vi "Safety_Check.vi"(1 "Adam Loop Count":i32, 2 "Ch Names":string[](array[string]), 3 "Values":dbl[](array[numeric]) format="%.2f") -> (0 "Scan comment":string)   [LabVIEW 2015]
uses:
  ADAM Client/Sub VIs/ADAM Controls/Update_scan_value.ctl
  Anemometry/Anemometry Sub Vis/Globals/Gas_management_global.vi
  ADAM_Global.vi
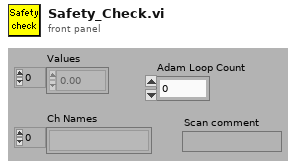
[diagram p1: front panel]
types:
  T1 = cluster{"Channel name":string, "Set value of A to":dbl, "Set value of B to":dbl, "Set value of C to":dbl, "Set value of D to":dbl}
  T2 = typedef "Update_scan_value.ctl" = cluster{"Channel Name":string, "New Value":dbl}
  T3 = enum16{"Append to Global", "Read Global then Clear"}
  T4 = enum16{"On", "Off", "Always On", "Always Off", "Delete"}
  T5 = typedef "LVDateTimeRec.ctl" = cluster{"fractional second":dbl, "second":i32, "minute":i32, "hour":i32, "day of month":i32, "month":i32, "year":i32, "day of week":i32, "day of year":i32, "DST":i32}
  T6 = cluster{"Channel name":string, "Set value of A to":dbl, "Set value of B to":dbl, "Set value of C to":dbl, "Set value of D to":dbl}[]
  T7 = typedef "Ch_description_ADAM.ctl" = cluster{"Ch Name":string, "Type":T8, "Function":T9, "Ch State":T10, "Calibration type":T11, "A":dbl, "B":dbl, "C":dbl, "D":dbl, "Comments":string, "Address":T12, "String":string, "Duty":u16}
  T8 = typedef "Module_type_ADAM.ctl" = string
  T9 = typedef "Function_ADAM.ctl" = enum16{"Analogue Input", "Digital Input", "Event counter", "Event rate", "Analogue Output", "Digital Output", "Relay Output"}
  T10 = typedef "Channel_State.ctl" = enum16{"On", "Off", "Always On", "Always Off"}
  T11 = typedef "Calib_type_ADAM.ctl" = enum16{"Raw", "Bx + A", "Cx^2 + Bx + A", "Dx^3 + Cx^2 + Bx + A", "In Band", "Hi-Tec Q", "Hi-Tec M_dot", "Text"}
  T12 = typedef "Address.ctl" = cluster{"Main":i32, "Ch.":i32, "Sub":i32, "Port Name":string}
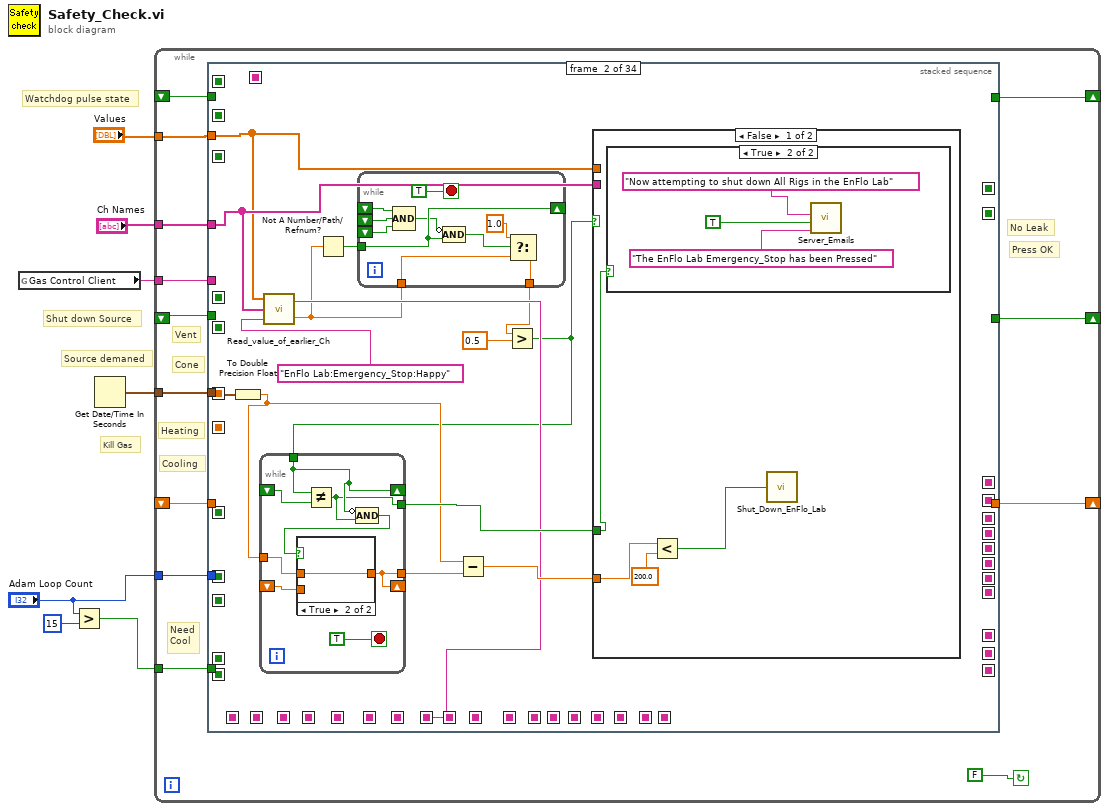
[diagram p0: block diagram]
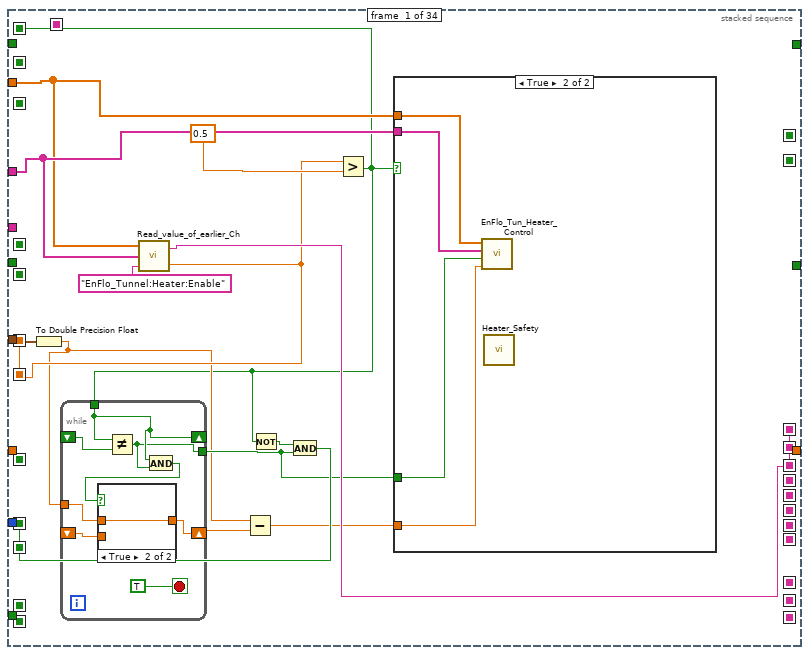
[diagram p2: hidden frame]
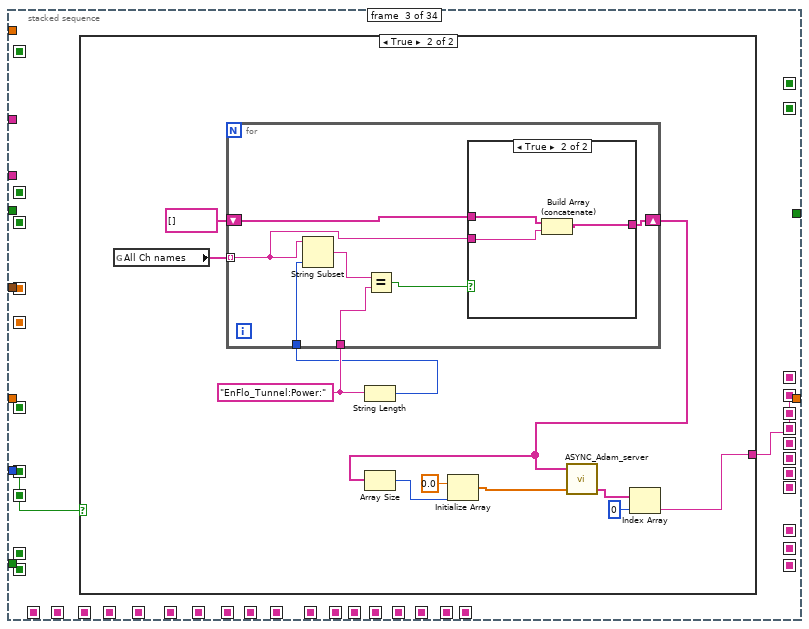
[diagram p8: hidden frame]
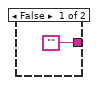
[diagram p9: hidden frame]
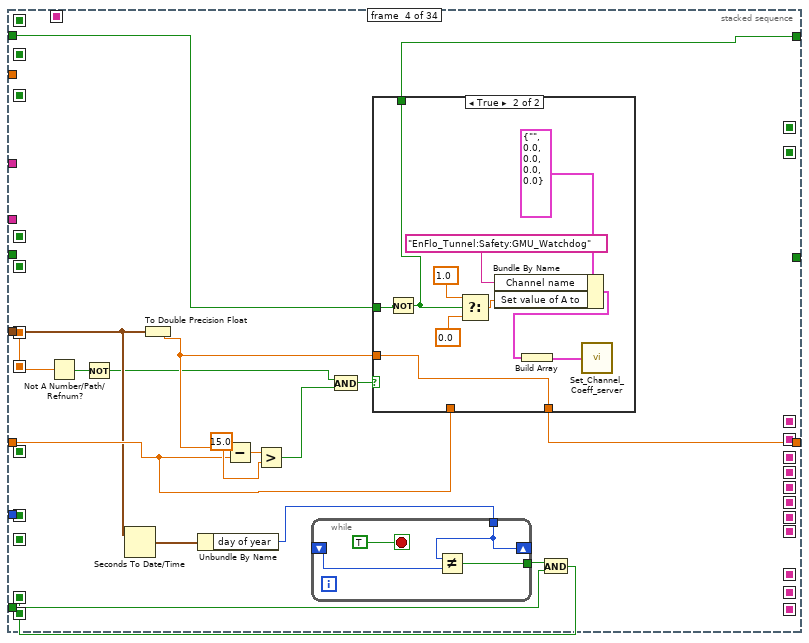
[diagram p11: hidden frame]
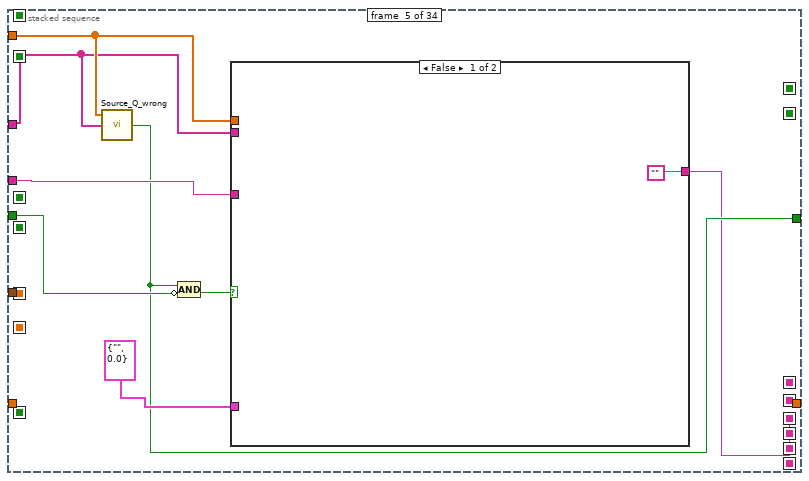
[diagram p13: hidden frame]
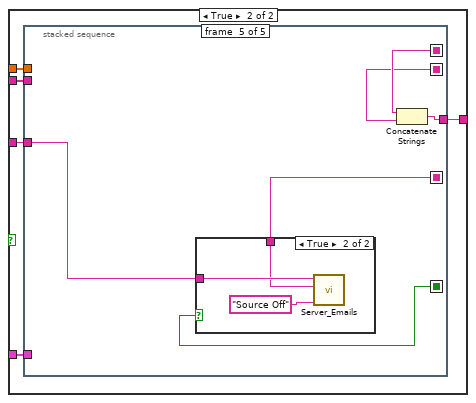
[diagram p14: hidden frame]
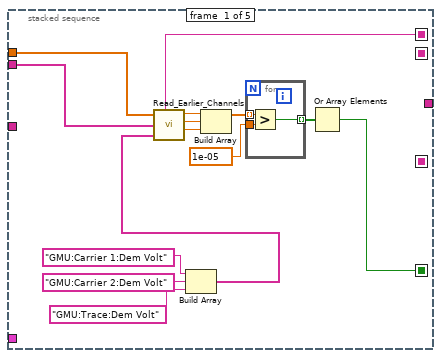
[diagram p15: hidden frame]
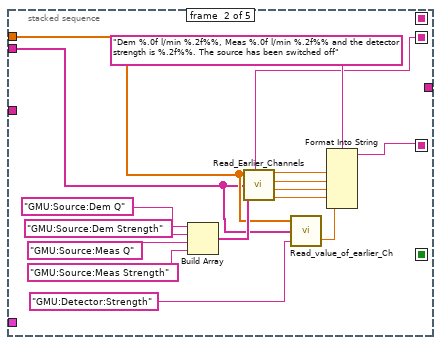
[diagram p16: hidden frame]
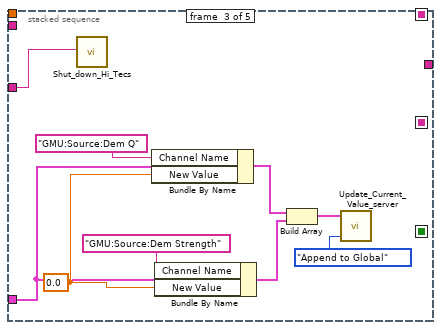
[diagram p17: hidden frame]
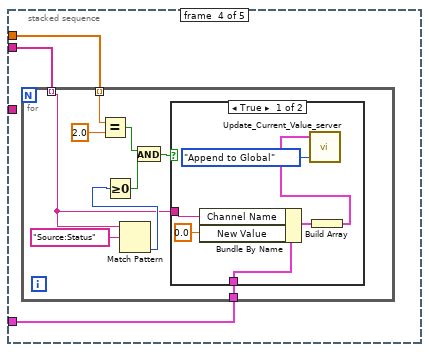
[diagram p18: hidden frame]
diagram:
  # "Shut down Source"
  # "Source demaned"
  # "Watchdog pulse state"
  # "Kill Gas"
  n1 = global read "Gas_management_global.vi" "Gas Control Client"() -> (w5:string)
  n2 = Greater?(x="Adam Loop Count", y=15) -> (0:w3:bool)
  n3 = Get Date/Time In Seconds() -> (seconds since 1Jan1904=w2:timestamp)
  n4 = while {
    shift-left: _ -> [w15]
    shift-right: [w14] -> _
    shift-left: _ -> [w17]
    shift-right: [w16] -> _
    tunnel: w5 -> [w19]
    tunnel: "Ch Names" -> [w20]
    tunnel: "Values" -> [w18]
    shift-right: [w12] -> _
    shift-left: _ -> [w11]
    tunnel: w3 -> [w10]
    tunnel: w2 -> [w9]
    tunnel: "Adam Loop Count" -> [w8]
    stop <- FALSE continue-if-true
    # "Need\nCool"
    # "Cooling"
    # "Heating"
    # "Cone"
    # "Vent"
    # "Press OK"
    # "No Leak"
    n5 = stacked-sequence {
      seq-local: [_ _ _ _ _ _ _ w272 _ _ _ _ _ _ _ _ _ _ _ _ _ _ _ _ _ _ _ _ _ _ _ _ _ _] -> [_ _ _ _ _ _ _ _ _ _ _ _ _ _ _ _ _ _ _ _ _ w692 _ _ _ _ _ _ _ _ _ _ _ _]
      seq-local: [w28 _ _ _ _ _ _ _ _ _ _ _ _ _ _ _ _ _ _ _ _ _ _ _ _ _ _ _ _ _ _ _ _ _] -> [_ _ w91 _ _ _ _ _ _ _ _ _ _ _ _ _ _ _ _ _ _ _ _ _ _ _ _ _ _ _ _ _ _ _]
      seq-local: [_ _ _ w121 _ _ _ _ _ _ _ _ _ _ _ _ _ _ _ _ _ _ _ _ _ _ _ _ _ _ _ _ _ _] -> [_ _ _ _ _ _ _ _ _ _ _ _ _ _ _ _ _ _ _ _ _ _ _ _ _ _ _ _ _ _ _ _ _ _]
      seq-local: [_ _ _ _ _ _ _ _ _ _ _ _ _ _ _ _ _ _ _ _ _ _ _ _ _ w822 _ _ _ _ _ _ _ _] -> [_ _ _ _ _ _ _ _ _ _ _ _ _ _ _ _ _ _ _ _ _ _ _ _ _ _ w834 _ _ _ _ _ _ _]
      seq-local: [_ _ _ _ _ _ _ _ _ _ _ _ _ _ _ _ _ _ _ _ _ _ _ _ _ _ w830 _ _ _ _ _ _ _] -> [_ _ _ _ _ _ _ _ _ _ _ _ _ _ _ _ _ _ _ _ _ _ _ _ _ _ _ _ _ _ _ w1016 _ _]
      seq-local: [w30 _ _ _ _ _ _ _ _ _ _ _ _ _ _ _ _ _ _ _ _ _ _ _ _ _ _ _ _ _ _ _ _ _] -> [_ _ _ _ _ _ _ _ _ _ _ _ _ _ _ _ _ _ _ _ _ _ _ _ _ _ _ _ _ _ _ _ _ w1096]
      seq-local: [_ _ w90 _ _ _ _ _ _ _ _ _ _ _ _ _ _ _ _ _ _ _ _ _ _ _ _ _ _ _ _ _ _ _] -> [_ _ _ _ _ _ _ _ _ _ _ _ _ _ _ _ _ _ _ _ _ _ _ _ _ _ _ _ _ _ _ _ _ w1095]
      seq-local: [_ _ _ _ w149 _ _ _ _ _ _ _ _ _ _ _ _ _ _ _ _ _ _ _ _ _ _ _ _ _ _ _ _ _] -> [_ _ _ _ _ _ _ _ _ _ _ _ _ _ _ _ _ _ _ _ _ _ _ _ _ _ _ _ _ _ _ _ _ w1094]
      seq-local: [_ _ _ _ _ w232 _ _ _ _ _ _ _ _ _ _ _ _ _ _ _ _ _ _ _ _ _ _ _ _ _ _ _ _] -> [_ _ _ _ _ _ _ _ _ _ _ _ _ _ _ _ _ _ _ _ _ _ _ _ _ _ _ _ _ _ _ _ _ w1093]
      seq-local: [_ _ _ _ _ _ w252 _ _ _ _ _ _ _ _ _ _ _ _ _ _ _ _ _ _ _ _ _ _ _ _ _ _ _] -> [_ _ _ _ _ _ _ _ _ _ _ _ _ _ _ _ _ _ _ _ _ _ _ _ _ _ _ _ _ _ _ _ _ w1092]
      seq-local: [_ _ _ _ _ _ _ w271 _ _ _ _ _ _ _ _ _ _ _ _ _ _ _ _ _ _ _ _ _ _ _ _ _ _] -> [_ _ _ _ _ _ _ _ _ _ _ _ _ _ _ _ _ _ _ _ _ _ _ _ _ _ _ _ _ _ _ _ _ w1091]
      seq-local: [_ _ _ _ _ _ _ _ _ _ _ w403 _ _ _ _ _ _ _ _ _ _ _ _ _ _ _ _ _ _ _ _ _ _] -> [_ _ _ _ _ _ _ _ _ _ _ _ _ _ _ _ _ _ _ _ _ _ _ _ _ _ _ _ _ _ _ _ _ w1090]
      seq-local: [_ _ _ _ _ _ _ _ _ _ _ _ w435 _ _ _ _ _ _ _ _ _ _ _ _ _ _ _ _ _ _ _ _ _] -> [_ _ _ _ _ _ _ _ _ _ _ _ _ _ _ _ _ _ _ _ _ _ _ _ _ _ _ _ _ _ _ _ _ w1081]
      seq-local: [_ _ _ _ _ _ _ _ _ _ _ _ _ _ _ _ _ w581 _ _ _ _ _ _ _ _ _ _ _ _ _ _ _ _] -> [_ _ _ _ _ _ _ _ _ _ _ _ _ _ _ _ _ _ _ _ _ _ _ _ _ _ _ _ _ _ _ _ _ w1080]
      seq-local: [_ _ _ _ _ _ _ _ _ _ _ _ _ _ _ _ _ _ _ _ _ w693 _ _ _ _ _ _ _ _ _ _ _ _] -> [_ _ _ _ _ _ _ _ _ _ _ _ _ _ _ _ _ _ _ _ _ _ _ _ _ _ _ _ _ _ _ _ _ w1083]
      seq-local: [_ _ _ _ _ _ _ _ _ _ _ _ _ _ _ _ _ _ _ _ _ _ w721 _ _ _ _ _ _ _ _ _ _ _] -> [_ _ _ _ _ _ _ _ _ _ _ _ _ _ _ _ _ _ _ _ _ _ _ _ _ _ _ _ _ _ _ _ _ w1084]
      seq-local: [_ _ _ _ _ _ _ _ _ _ _ _ _ _ _ _ _ _ _ _ _ _ _ _ _ w816 _ _ _ _ _ _ _ _] -> [_ _ _ _ _ _ _ _ _ _ _ _ _ _ _ _ _ _ _ _ _ _ _ _ _ _ _ _ _ _ _ _ _ w1085]
      seq-local: [_ _ _ _ _ _ _ _ _ _ _ _ _ _ _ _ _ _ _ _ _ _ _ _ _ _ w827 _ _ _ _ _ _ _] -> [_ _ _ _ _ _ _ _ _ _ _ _ _ _ _ _ _ _ _ _ _ _ _ _ _ _ _ _ _ _ _ _ _ w1086]
      seq-local: [_ _ _ _ _ _ _ _ _ _ _ _ _ w466 _ _ _ _ _ _ _ _ _ _ _ _ _ _ _ _ _ _ _ _] -> [_ _ _ _ _ _ _ _ _ _ _ _ _ _ _ _ _ _ _ _ _ _ _ _ _ _ _ _ _ _ _ _ _ w1087]
      seq-local: [_ _ _ _ _ _ _ _ _ _ _ _ _ _ _ _ _ _ _ _ _ _ _ _ _ _ _ _ _ _ w972 _ _ _] -> [_ _ _ _ _ _ _ _ _ _ _ _ _ _ _ _ _ _ _ _ _ _ _ _ _ _ _ _ _ _ _ _ _ w1088]
      seq-local: [_ _ _ _ _ _ _ _ _ _ _ _ _ _ _ _ _ _ _ _ _ _ _ _ _ _ _ _ _ _ _ w1014 _ _] -> [_ _ _ _ _ _ _ _ _ _ _ _ _ _ _ _ _ _ _ _ _ _ _ _ _ _ _ _ _ _ _ _ _ w1089]
      seq-local: [w29 _ _ _ _ _ _ _ _ _ _ _ _ _ _ _ _ _ _ _ _ _ _ _ _ _ _ _ _ _ _ _ _ _] -> [_ _ _ w119 _ _ _ _ _ _ _ _ _ _ _ _ _ _ _ _ _ _ _ _ _ _ _ w904 w931 _ _ _ _ _]
      seq-local: [_ _ _ _ _ _ _ _ w290 _ _ _ _ _ _ _ _ _ _ _ _ _ _ _ _ _ _ _ _ _ _ _ _ _] -> [_ _ _ _ _ _ _ _ _ _ _ _ _ _ _ _ _ _ _ _ _ w691 _ _ _ _ _ _ _ _ _ _ _ _]
      seq-local: [_ _ _ _ _ _ _ _ w289 _ _ _ _ _ _ _ _ _ _ _ _ _ _ _ _ _ _ _ _ _ _ _ _ _] -> [_ _ _ _ _ _ _ _ _ _ _ _ _ _ _ _ _ _ _ _ _ _ _ _ _ _ _ _ _ _ _ _ _ w1079]
      seq-local: [_ _ _ _ _ _ _ _ w288 _ _ _ _ _ _ _ _ _ _ _ _ _ _ _ _ _ _ _ _ _ _ _ _ _] -> [_ _ _ _ _ _ _ _ _ w317 w336 _ _ _ _ _ _ _ _ _ _ _ _ _ _ w817 w826 _ _ w957 _ _ _ _]
      seq-local: [_ _ _ _ _ _ _ _ _ _ w333 _ _ _ _ _ _ _ _ _ _ _ _ _ _ _ _ _ _ _ _ _ _ _] -> [_ _ _ _ _ _ _ _ _ _ _ _ _ _ _ _ _ _ _ _ _ _ _ _ _ _ _ _ _ _ _ _ _ w1077]
      seq-local: [_ _ _ _ _ _ _ _ _ _ _ _ _ _ _ _ w535 _ _ _ _ _ _ _ _ _ _ _ _ _ _ _ _ _] -> [_ _ _ _ _ _ _ _ _ _ _ _ _ _ _ _ _ _ _ _ _ _ _ _ _ _ _ _ _ _ _ _ _ w1078]
      seq-local: [_ _ _ _ _ _ _ _ _ _ _ _ _ _ _ _ _ _ _ _ _ _ _ _ w784 _ _ _ _ _ _ _ _ _] -> [_ _ _ _ _ _ _ _ _ _ _ _ _ _ _ _ _ _ _ _ _ _ _ _ _ _ _ _ _ _ _ _ _ w1076]
      seq-local: [_ _ _ _ _ _ _ _ _ _ _ _ _ _ w494 _ _ _ _ _ _ _ _ _ _ _ _ _ _ _ _ _ _ _] -> [_ _ _ _ _ _ _ _ _ _ _ _ _ _ _ _ _ _ _ _ _ _ _ _ _ _ _ _ _ _ _ _ _ w1075]
      seq-local: [_ w55 _ _ _ _ _ _ _ _ _ _ _ _ _ _ _ _ _ _ _ _ _ _ _ _ _ _ _ _ _ _ _ _] -> [_ _ _ _ _ _ _ _ _ _ _ _ _ _ _ _ _ _ _ _ _ _ _ _ _ _ _ _ _ _ _ _ _ w1074]
      seq-local: [_ _ _ _ _ _ _ _ _ _ _ _ _ _ _ _ _ _ _ _ _ _ _ _ _ _ _ _ _ _ _ _ w1040 _] -> [_ _ _ _ _ _ _ _ _ _ _ _ _ _ _ _ _ _ _ _ _ _ _ _ _ _ _ _ _ _ _ _ _ w1073]
      seq-local: [_ _ _ _ _ _ _ _ _ _ _ _ _ _ _ _ _ _ w603 _ _ _ _ _ _ _ _ _ _ _ _ _ _ _] -> [_ _ _ _ _ _ _ _ _ _ _ _ _ _ _ _ _ _ _ _ _ _ _ _ _ _ _ _ _ _ _ _ _ w1071]
      seq-local: [_ _ _ _ _ _ _ _ _ _ _ _ _ _ _ _ _ _ _ _ w671 _ _ _ _ _ _ _ _ _ _ _ _ _] -> [_ _ _ _ _ _ _ _ _ _ _ _ _ _ _ _ _ _ _ _ _ _ _ _ _ _ _ _ _ _ _ _ _ w1072]
      seq-local: [w21 _ _ _ _ _ _ _ _ _ _ _ _ _ _ _ _ _ _ _ _ _ _ _ _ _ _ _ _ _ _ _ _ _] -> [_ _ _ _ _ _ _ _ _ _ _ _ _ _ _ _ _ _ _ _ _ _ w720 w741 _ _ _ _ _ _ _ _ _ _]
      seq-local: [_ _ _ _ _ _ _ _ _ _ _ _ _ _ _ _ _ _ _ _ _ _ _ w739 _ _ _ _ _ _ _ _ _ _] -> [_ _ _ _ _ _ _ _ _ _ _ _ _ _ _ _ _ _ _ _ _ _ _ _ _ _ _ _ _ _ _ _ _ w1070]
      seq-local: [_ _ _ _ _ _ _ _ _ _ _ _ _ _ _ _ _ _ _ _ _ _ _ _ _ _ _ _ _ w956 _ _ _ _] -> [_ _ _ _ _ _ _ _ _ _ _ _ _ _ _ _ _ _ _ _ _ _ _ _ _ _ _ _ _ _ _ _ _ w1069]
      seq-local: [_ _ _ _ _ _ _ _ _ _ _ _ _ w455 _ _ _ _ _ _ _ _ _ _ _ _ _ _ _ _ _ _ _ _] -> [_ _ _ _ _ _ _ _ _ _ _ _ _ _ _ w515 _ _ _ _ _ _ _ _ _ _ _ _ _ _ _ _ _ _]
      seq-local: [_ _ _ _ _ _ _ _ _ _ _ _ _ _ w493 _ _ _ _ _ _ _ _ _ _ _ _ _ _ _ _ _ _ _] -> [_ _ _ _ _ _ _ _ _ _ _ _ _ _ _ w516 _ _ _ _ _ _ _ _ _ _ _ _ _ _ _ _ _ _]
      seq-local: [_ _ _ _ _ _ _ _ _ _ _ _ _ _ _ _ _ _ _ _ _ _ _ _ _ _ w825 _ _ _ _ _ _ _] -> [_ _ _ _ _ _ _ _ _ _ _ _ _ _ _ _ _ _ _ _ _ _ _ _ _ _ _ w902 w921 _ _ _ _ _]
      seq-local: [_ _ _ _ _ _ _ _ _ _ _ _ _ _ _ _ _ _ _ _ _ _ _ _ _ _ _ w896 _ _ _ _ _ _] -> [_ _ _ _ _ _ _ _ _ _ _ _ _ _ _ _ _ _ _ _ _ _ _ _ _ _ _ _ _ _ _ _ _ w1068]
      seq-local: [_ _ _ _ _ _ _ _ _ _ _ _ _ _ _ _ _ _ _ _ _ _ _ _ _ _ _ _ w922 _ _ _ _ _] -> [_ _ _ _ _ _ _ _ _ _ _ _ _ _ _ _ _ _ _ _ _ _ _ _ _ _ _ _ _ _ _ _ _ w1067]
      seq-local: [_ _ _ _ _ _ _ _ _ w318 _ _ _ _ _ _ _ _ _ _ _ _ _ _ _ _ _ _ _ _ _ _ _ _] -> [_ _ _ _ _ _ _ _ _ _ w332 _ _ _ _ _ _ _ _ _ _ _ _ _ _ _ _ _ _ _ _ _ _ _]
      seq-local: [_ _ _ _ _ _ _ _ _ _ _ _ _ _ _ _ _ _ w602 _ _ _ _ _ _ _ _ _ _ _ _ _ _ _] -> [_ _ _ _ _ _ _ _ _ _ _ _ _ _ _ _ _ _ _ w641 _ _ _ _ _ _ _ _ _ _ _ _ _ _]
      seq-local: [_ _ _ _ _ _ _ _ _ _ _ _ _ _ _ _ _ _ _ w635 _ _ _ _ _ _ _ _ _ _ _ _ _ _] -> [_ _ _ _ _ _ _ _ _ _ _ _ _ _ _ _ _ _ _ _ _ _ _ _ _ _ _ _ _ _ _ _ _ w1066]
      tunnel: w20 -> [w32 w61 _ _ w151 w239 w254 w273 w291 w319 w334 w404 w436 w465 w495 _ w536 w583 w605 w647 w673 w694 w725 w745 w778 w820 w835 w889 _ _ w975 _ _ _]
      tunnel: w19 -> [_ _ _ _ w156 _ w253 _ _ _ _ _ _ _ _ _ _ _ _ _ _ _ _ _ _ _ _ _ _ _ _ _ _ _]
      tunnel: w18 -> [w31 w60 _ _ w152 w235 w255 w274 w292 w320 w335 w405 w437 w463 w496 _ w537 w584 w606 w648 w674 w695 w726 w746 w777 w821 w836 w890 _ _ w976 _ _ _]
      tunnel: w17 -> [_ _ _ w132 _ _ _ _ _ _ _ _ _ _ _ _ _ _ _ _ _ _ _ _ _ _ _ _ _ _ _ _ _ _]
      tunnel: [_ _ _ w131 _ _ _ _ _ _ _ _ _ _ _ _ _ _ _ _ _ _ _ _ _ _ _ _ _ _ _ _ _ _] -> w16
      tunnel: w15 -> [_ _ _ _ w155 _ _ _ _ _ _ _ _ _ _ _ _ _ _ _ _ _ _ _ _ _ _ _ _ _ _ _ _ _]
      tunnel: [_ _ _ _ w150 _ _ _ _ _ _ _ _ _ _ _ _ _ _ _ _ _ _ _ _ _ _ _ _ _ _ _ _ _] -> w14
      tunnel: [_ _ _ w130 _ _ _ _ _ _ _ _ _ _ _ _ _ _ _ _ _ _ _ _ _ _ _ _ _ _ _ _ _ _] -> w12
      tunnel: w11 -> [_ _ _ w126 _ _ _ _ _ _ _ _ _ _ _ _ _ _ _ _ _ _ _ _ _ _ _ _ _ _ _ _ _ _]
      tunnel: w10 -> [_ _ _ w122 _ _ _ _ _ _ _ _ _ w467 _ _ w533 w582 w604 w645 w672 _ _ _ _ _ w831 w897 w927 w955 _ w1015 _ _]
      tunnel: w9 -> [w25 w58 _ w120 _ _ _ _ _ _ _ _ _ _ _ _ w534 _ _ _ _ _ _ _ _ _ _ _ _ _ _ _ _ _]
      tunnel: w8 -> [_ _ _ _ _ _ _ _ _ _ _ _ _ _ _ _ _ _ _ _ _ _ _ _ _ _ _ _ _ _ _ _ w1052 _]
      frame #0 {
        n6 = To Double Precision Float(number=w25) -> (double precision float=w24:dbl)
        n7 = call "Read_value_of_earlier_Ch.vi"("Desired Ch to Read"="EnFlo_Tunnel:Heater:Enable", "Ch names"=w32, "Present scan array"=w31) -> ("Value"=w29:dbl, "Scan comment"=w30:string)  [unwired: 1 in]
        n8 = Greater?(x=w29, y=0.5) -> (0:w21:bool)
        n9 = while {
          shift-right: [w40] -> _
          shift-left: _ -> [w42]
          tunnel: w21 -> [w40]
          tunnel: [w39] -> w26
          shift-right: [w37] -> w23
          shift-left: _ -> [w35]
          tunnel: w24 -> [w36]
          stop <- TRUE stop-if-true
          n10 = Not Equal?(x=w40, y=w42) -> (x != y?=w39:bool)
          n11 = And(x=w40, y=w39) -> (x .and. y?=w38:bool)
          n12 = case shown="True" w38 {
            tunnel: [w43 w44] -> w37
            tunnel: w36 -> [_ w44]
            tunnel: w35 -> [w43 _]
            frame False {
            }
            frame True {
            }
          }
        }
        n13 = Subtract(x=w24, y=w23) -> (x-y=w22:dbl)
        n14 = Not(x=w21) -> (.not. x?=w27:bool)
        n15 = And(x=w27, y=w26) -> (x .and. y?=w28:bool)
        n16 = case shown="True" w21 {
          tunnel: w31 -> [_ w48]
          tunnel: w32 -> [_ w47]
          tunnel: w26 -> [_ w46]
          tunnel: w22 -> [_ w45]
          frame False {
          }
          frame True {
            n17 = call "EnFlo_Tun_Heater_Control.vi"("Heaters Enabled time (s)"=w45, "Heaters Just Enabled"=w46, "Ch Names"=w47, "Values"=w48) -> ()  [unwired: 1 in]
            n18 = call "Heater_Safety.vi"() -> ()  [unwired: 3 in, 5 out]
          }
        }
      }
      frame #1 {
        n19 = To Double Precision Float(number=w58) -> (double precision float=w57:dbl)
        n20 = call "Read_value_of_earlier_Ch.vi"("Desired Ch to Read"="EnFlo Lab:Emergency_Stop:Happy", "Ch names"=w61, "Present scan array"=w60) -> ("Value"=w53:dbl, "Scan comment"=w55:string)  [unwired: 1 in]
        n21 = Not A Number/Path/Refnum?(number/path/refnum=w53) -> (NaN/Path/Refnum?=w52:bool)
        n22 = while {
          tunnel: w53 -> [w65]
          shift-right: [w69] -> _
          shift-left: _ -> [w72]
          tunnel: w52 -> [w69]
          shift-left: _ -> [w71]
          shift-left: _ -> [w70]
          tunnel: [w64] -> w49
          stop <- TRUE stop-if-true
          n23 = Compound Arithmetic op=AND(w72, w71, w70) -> (w68:bool)
          n24 = Compound Arithmetic op=AND(invert w68, w69) -> (w67:bool)
          n25 = Select(t=1.0, s=w67, f=w65) -> (s? t:f=w64:dbl)
        }
        n26 = Greater?(x=w49, y=0.5) -> (0:w50:bool)
        n27 = while {
          shift-right: [w78] -> _
          shift-left: _ -> [w80]
          tunnel: w50 -> [w78]
          tunnel: [w77] -> w59
          shift-right: [w73] -> _
          shift-left: _ -> [w74]
          tunnel: w57 -> [w75]
          tunnel: [w73] -> w54
          stop <- TRUE stop-if-true
          n28 = Not Equal?(x=w78, y=w80) -> (x != y?=w77:bool)
          n29 = Compound Arithmetic op=AND(invert w78, w77) -> (w76:bool)
          n30 = case shown="True" w76 {
            tunnel: [w81 w82] -> w73
            tunnel: w75 -> [_ w82]
            tunnel: w74 -> [w81 _]
            frame False {
            }
            frame True {
            }
          }
        }
        n31 = Subtract(x=w57, y=w54) -> (x-y=w56:dbl)
        n32 = case shown="False" w50 {
          tunnel: w60 -> [_ _]
          tunnel: w61 -> [_ _]
          tunnel: w59 -> [w84 _]
          tunnel: w56 -> [w86 _]
          frame False {
            n33 = case shown="True" w84 {
              frame False {
              }
              frame True {
                n34 = call "Server_Emails.vi"("Message"="Now attempting to shut down All Rigs in the EnFlo Lab", "Contact All clients?"=TRUE, "Subject"="The EnFlo Lab Emergency_Stop has been Pressed") -> ()  [unwired: 2 in, 3 out]
              }
            }
            n35 = Less?(x=w86, y=200.0) -> (x < y?=w83:bool)
            n36 = call "Shut_Down_EnFlo_Lab.vi"("Initial Shutdown"=w83) -> ()
          }
          frame True {
          }
        }
      }
      frame #2 {
        n37 = case shown="True" w91 {
          tunnel: ["" w94] -> w90
          frame False {
          }
          frame True {
            w103 = "EnFlo_Tunnel:Power:"
            n38 = global read "ADAM_Global.vi" "All Ch names"() -> (w93:string[])
            n39 = String Length(string=w103) -> (length=w102:i32)
            n40 = for {
              shift-right: [w105] -> w98
              shift-left: string[] [] -> [w106]
              tunnel: w93 -> [w109] mode=indexing
              tunnel: w102 -> [w110]
              tunnel: w103 -> [w107]
              n41 = String Subset(string=w109, length (rest)=w110) -> (substring=w108:string)  [unwired: 1 out]
              n42 = Equal?(x=w108, y=w107) -> (x = y?=w104:bool)
              n43 = case shown="True" w104 {
                tunnel: w109 -> [_ w114]
                tunnel: w106 -> [w111 w112]
                tunnel: [w111 w113] -> w105
                frame False {
                }
                frame True {
                  n44 = Build Array (concatenate)(w112, w114) -> (w113:string[])
                }
              }
            }
            n45 = Array Size(array=w98) -> (size(s)=w99:i32)
            n46 = Initialize Array(0.0 ("element"), w99) -> (w97:dbl[])
            n47 = call "ASYNC_Adam_server.vi"("Values"=w97, "Channel Names"=w98) -> ("Scan Comments"=w96:string[])  [unwired: 1 in, 2 out]
            n48 = Index Array(array=w96, index=0) -> (element=w94:string)
          }
        }
      }
      frame #3 {
        n49 = Not A Number/Path/Refnum?(number/path/refnum=w119) -> (NaN/Path/Refnum?=w118:bool)
        n50 = Not(x=w118) -> (.not. x?=w116:bool)
        n51 = Seconds To Date/Time(time stamp (now)=w120) -> (date time rec=w125:T5)  [unwired: 1 in]
        n52 = To Double Precision Float(number=w120) -> (double precision float=w129:dbl)
        n53 = Unbundle By Name(w125) -> ("day of year"=w124:i32)
        n54 = Subtract(x=w129, y=w126) -> (x-y=w128:dbl)
        n55 = Greater?(x=w128, y=15.0) -> (0:w117:bool)
        n56 = while {
          shift-right: [w136] -> _
          shift-left: _ -> [w135]
          tunnel: w124 -> [w136]
          tunnel: [w134] -> w123
          stop <- TRUE stop-if-true
          n57 = Not Equal?(x=w136, y=w135) -> (x != y?=w134:bool)
        }
        n58 = And(x=w116, y=w117) -> (x .and. y?=w115:bool)
        n59 = case shown="True" w115 {
          tunnel: w132 -> [w137 w141]
          tunnel: [w137 w140] -> w131
          tunnel: [w138 w139] -> w130
          tunnel: w129 -> [_ w139]
          tunnel: w126 -> [w138 _]
          frame False {
          }
          frame True {
            n60 = Not(x=w141) -> (.not. x?=w140:bool)
            n61 = Select(t=1.0 ("Suction"), s=w140, f=0.0 ("Suction")) -> (s? t:f=w144:dbl)
            n62 = Bundle By Name(cluster=T1 {"Channel name"="", "Set value of A to"=0.0, "Set value of B to"=0.0, "Set value of C to"=0.0, "Set value of D to"=0.0}, "Channel name"="EnFlo_Tunnel:Safety:GMU_Watchdog" ("Desired Ch to Read"), "Set value of A to"=w144) -> (w148:T1)
            n63 = Build Array(w148) -> (w143:T6)
            n64 = call "Set_Channel_Coeff_server.vi"("Set Array"=w143) -> ()
          }
        }
        n65 = And(x=w123, y=w122) -> (x .and. y?=w121:bool)
      }
      frame #4 {
        n66 = call "Source_Q_wrong.vi"("Ch Names"=w151, "Values"=w152) -> ("Gas Error?"=w150:bool)  [unwired: 1 out]
        n67 = Compound Arithmetic op=AND(w150, invert w155) -> (w154:bool)
        n68 = case shown="False" w154 {
          tunnel: w156 -> [_ w162]
          tunnel: w152 -> [_ w161]
          tunnel: w151 -> [_ w160]
          tunnel: T2 {"Channel Name"="", "New Value"=0.0} ("Update Scan Value Cluster") -> [_ w159]
          tunnel: ["" w158] -> w149
          frame False {
          }
          frame True {
            n69 = stacked-sequence {
              seq-local: [_ w194 _ _ _] -> [_ _ _ _ w227]
              seq-local: [w164 _ _ _ _] -> [_ _ _ _ w226]
              seq-local: [w163 _ _ _ _] -> [_ _ _ _ w225]
              seq-local: [_ w180 _ _ _] -> [_ _ _ _ w224]
              tunnel: w162 -> [_ _ w197 _ w228]
              tunnel: w161 -> [w174 w184 _ w206 _]
              tunnel: w160 -> [w175 w183 _ w207 _]
              tunnel: w159 -> [_ _ w196 w205 _]
              tunnel: [_ _ _ _ w223] -> w158
              frame #0 {
                n70 = Build Array("GMU:Carrier 1:Dem Volt", "GMU:Carrier 2:Dem Volt", "GMU:Trace:Dem Volt") -> (w176:string[])
                n71 = call "Read_Earlier_Channels.vi"("Present scan array"=w174, "Ch names"=w175, "Desired Channels"=w176) -> ("Scan comments"=w163:string, "Index 0"=w170:dbl, "Index 1"=w169:dbl, "Index 2"=w168:dbl)  [unwired: 2 out]
                n72 = Build Array(w170, w169, w168) -> (w167:dbl[])
                n73 = for {
                  tunnel: w167 -> [w179] mode=indexing
                  tunnel: 1e-05 -> [w178]
                  tunnel: [w177] -> w165 mode=indexing
                  n74 = Greater?(x=w179, y=w178) -> (0:w177:bool)
                }
                n75 = Or Array Elements(Boolean array=w165) -> (logical OR=w164:bool)
              }
              frame #1 {
                n76 = Build Array("GMU:Source:Dem Q", "GMU:Source:Dem Strength", "GMU:Source:Meas Q", "GMU:Source:Meas Strength") -> (w189:string[])
                n77 = call "Read_Earlier_Channels.vi"("Present scan array"=w184, "Ch names"=w183, "Desired Channels"=w189) -> ("Scan comments"=w180:string, "Index 0"=w188:dbl, "Index 1"=w187:dbl, "Index 2"=w186:dbl, "Index 3"=w185:dbl)  [unwired: 1 out]
                n78 = call "Read_value_of_earlier_Ch.vi"("Desired Ch to Read"="GMU:Detector:Strength", "Ch names"=w183, "Present scan array"=w184) -> ("Value"=w181:dbl)  [unwired: 1 in, 1 out]
                n79 = Format Into String(format string="Dem %.0f l/min %.2f%%, Meas %.0f l/min %.2f%% and the detector strength is %.2f%%. The source has been switched off" ("Format String"), w188, w187, w186, w185, w181) -> (resulting string=w194:string)  [unwired: 2 in, 1 out]
              }
              frame #2 {
                w198 = 0.0 ("Bundle Element")
                n80 = call "Shut_down_Hi_Tecs.vi"("Client Name"=w197) -> ()  [unwired: 6 out]
                n81 = Bundle By Name(cluster=w196, "Channel Name"="GMU:Source:Dem Q", "New Value"=w198) -> (w203:T2)
                n82 = Bundle By Name(cluster=w196, "Channel Name"="GMU:Source:Dem Strength", "New Value"=w198) -> (w204:T2)
                n83 = Build Array(w203, w204) -> (w200:T2[])
                n84 = call "Update_Current_Value_server.vi"("Mode"=T3."Append to Global", "Update array in"=w200) -> ()  [unwired: 1 in, 1 out]
              }
              frame #3 {
                n85 = for {
                  tunnel: w207 -> [w208] mode=indexing
                  tunnel: w206 -> [w214] mode=indexing
                  tunnel: w205 -> [w209]
                  n86 = Equal?(x=w214, y=2.0) -> (x = y?=w211:bool)
                  n87 = Match Pattern(string=w208, regular expression="Source:Status") -> (offset past match=w215:i32)  [unwired: 4 out]
                  n88 = Greater Or Equal To 0?(x=w215) -> (x >= 0?=w212:bool)
                  n89 = And(x=w211, y=w212) -> (x .and. y?=w210:bool)
                  n90 = case shown="True" w210 {
                    tunnel: w209 -> [w222 _]
                    tunnel: w208 -> [w221 _]
                    frame True {
                      n91 = Bundle By Name(cluster=w222, "Channel Name"=w221, "New Value"=0.0) -> (w219:T2)
                      n92 = Build Array(w219) -> (w218:T2[])
                      n93 = call "Update_Current_Value_server.vi"("Mode"=T3."Append to Global", "Update array in"=w218) -> ()  [unwired: 1 in, 1 out]
                    }
                    frame False {
                    }
                  }
                }
              }
              frame #4 {
                n94 = case shown="True" w226 {
                  tunnel: w228 -> [_ w231]
                  tunnel: w227 -> [_ w230]
                  frame False {
                  }
                  frame True {
                    n95 = call "Server_Emails.vi"("Client Name Contains"=w231, "Message"=w230, "Subject"="Source Off") -> ()  [unwired: 2 in, 3 out]
                  }
                }
                n96 = Concatenate Strings(w225, w224) -> (w223:string)
              }
            }
          }
        }
      }
      frame #5 {
        n97 = global read "ADAM_Global.vi" "Program Hung Clients"() -> (w240:string[])
        n98 = for {
          tunnel: w240 -> [w249] mode=indexing
          tunnel: w235 -> [w251]
          tunnel: w239 -> [w250]
          tunnel: [w247] -> w238 mode=indexing
          tunnel: [w244] -> w237 mode=indexing
          shift-right: [w242] -> w232
          shift-left: "" -> [w243]
          n99 = call "Split_Ch_name.vi"("Ch name"=w249) -> ("Low level"=w246:string)  [unwired: 2 out]
          n100 = call "Shut_Down_Client_Demands.vi"("Ch Names"=w250, "Values"=w251, "Client Name"=w249) -> ("Comments"=w241:string)
          n101 = Concatenate Strings(w243, w241) -> (w242:string)
          n102 = Concatenate Strings(w246, ":Source:Status") -> (w247:string)
          n103 = Concatenate Strings(w246, ":Program:Sync") -> (w244:string)
        }
        n104 = Build Array (concatenate)(w238, w237) -> (w236:string[])
        n105 = call "Cntrl_Ch_Status_low.vi"("Mode"=T4."Delete", "Channel names"=w236) -> ()  [unwired: 1 out]
      }
      frame #6 {
        n106 = while {
          tunnel: w255 -> [w267]
          tunnel: w254 -> [w266]
          shift-right: [w261] -> _
          shift-left: _ -> [w262]
          tunnel: w253 -> [w259]
          tunnel: [w257] -> w252
          stop <- FALSE continue-if-true
          n107 = call "Read_value_of_earlier_Ch.vi"("Desired Ch to Read"="GMU:Detector:Happy", "Ch names"=w266, "Present scan array"=w267) -> ("Value"=w264:dbl, "Scan comment"=w257:string)  [unwired: 1 in]
          n108 = Greater?(x=w264, y=0.5) -> (0:w261:bool)
          n109 = Compound Arithmetic op=AND(invert w261, w262) -> (w260:bool)
          n110 = case shown="True" w260 {
            tunnel: w259 -> [_ w269]
            frame False {
            }
            frame True {
              n111 = call "Server_Emails.vi"("Client Name Contains"=w269, "Message"="The GMU Gas detector IR2100 is unhappy. Please check concentrations etc. This will have turned off the gases from the outside bottle store.  You will need to repress the blue gas button after clearing the fault by purging the source with carrier gas only.", "Subject"="GMU Gas Detector Unhappy") -> ()  [unwired: 2 in, 3 out]
            }
          }
        }
        n112 = global write "ADAM_Global.vi" "Program Hung Clients"(string[] [] ("Program Hung Clients")) -> ()
      }
      frame #7 {
        n113 = while {
          tunnel: w274 -> [w284]
          tunnel: w273 -> [w283]
          shift-right: [w278] -> w272
          shift-left: _ -> [w279]
          tunnel: [w275] -> w271
          stop <- FALSE continue-if-true
          n114 = call "Read_value_of_earlier_Ch.vi"("Desired Ch to Read"="EnFlo Lab:Leak_Detector:Happy", "Ch names"=w283, "Present scan array"=w284) -> ("Value"=w281:dbl, "Scan comment"=w275:string)  [unwired: 1 in]
          n115 = Greater?(x=w281, y=0.5) -> (0:w278:bool)
          n116 = Compound Arithmetic op=AND(invert w278, w279) -> (w277:bool)
          n117 = case shown="True" w277 {
            frame False {
            }
            frame True {
              n118 = call "Server_Emails.vi"("Client Name Contains"="EnFlo_Tunnel", "Message"="The leak detector is indicating a leak under the Enflo Tunnel. The chiller pumps should automaticaly be turned off and the cooling circuit isolated from the  University Chilled water system. The heaters should also have been disabled.", "Subject"="Leak Detected under EnFlo Tunnel") -> ()  [unwired: 2 in, 3 out]
            }
          }
        }
      }
      frame #8 {
        n119 = while {
          tunnel: w292 -> [w298]
          tunnel: w291 -> [w297]
          shift-right: [w309] -> w290
          shift-left: _ -> [w310]
          tunnel: [w301] -> w289
          tunnel: [w293] -> w288
          stop <- FALSE continue-if-true
          n120 = call "Read_value_of_earlier_Ch.vi"("Desired Ch to Read"="EnFlo_Tunnel:Chiller_Pump:Enable", "Ch names"=w297, "Present scan array"=w298) -> ("Value"=w304:dbl, "Scan comment"=w302:string)  [unwired: 1 in]
          n121 = call "Read_value_of_earlier_Ch.vi"("Desired Ch to Read"="EnFlo_Tunnel:Chilled Water:Pressure_OK", "Ch names"=w297, "Present scan array"=w298) -> ("Value"=w312:dbl, "Scan comment"=w303:string)  [unwired: 1 in]
          n122 = call "Read_value_of_earlier_Ch.vi"("Desired Ch to Read"="EnFlo_Tunnel:Chiller_Pump:Running", "Ch names"=w297, "Present scan array"=w298) -> ("Value"=w295:dbl, "Scan comment"=w294:string)  [unwired: 1 in]
          n123 = Greater?(x=w312, y=0.5) -> (0:w309:bool)
          n124 = Greater?(x=w304, y=0.5) -> (0:w300:bool)
          n125 = Compound Arithmetic op=AND(invert w309, w310, w300) -> (w308:bool)
          n126 = case shown="True" w308 {
            frame False {
            }
            frame True {
              n127 = call "Server_Emails.vi"("Client Name Contains"="EnFlo_Tunnel", "Message"="The pressure in the chilled water  for the Enflo Tunnel has tripped the system. The chiller pumps should automaticaly be turned off and the cooling circuit isolated from the  University Chilled water system. The heaters should also have been disabled.", "Subject"="EnFlo Chilled Water Overpressure Trip") -> ()  [unwired: 2 in, 3 out]
            }
          }
          n128 = Greater?(x=w295, y=0.5) -> (0:w293:bool)
          n129 = Concatenate Strings(w302, w303, w294) -> (w301:string)
        }
      }
      frame #9 {
        n130 = case shown="True" w317 {
          tunnel: w320 -> [_ w328]
          tunnel: w319 -> [_ w327]
          tunnel: [FALSE w322] -> w318
          frame False {
          }
          frame True {
            n131 = call "Read_value_of_earlier_Ch.vi"("Desired Ch to Read"="EnFlo_Tunnel:Floor_Cooling:Enable", "Ch names"=w327, "Present scan array"=w328) -> ("Value"=w330:dbl)  [unwired: 1 in, 1 out]
            n132 = call "Read_value_of_earlier_Ch.vi"("Desired Ch to Read"="EnFlo_Tunnel:Heat_Ex_Div_Valve:Dem Pos", "Ch names"=w327, "Present scan array"=w328) -> ("Value"=w325:dbl)  [unwired: 1 in, 1 out]
            n133 = Greater Than 0?(x=w325) -> (x > 0?=w323:bool)
            n134 = Greater?(x=w330, y=0.5) -> (0:w324:bool)
            n135 = Or(x=w324, y=w323) -> (x .or. y?=w322:bool)
          }
        }
      }
      frame #10 {
        n136 = case shown="True" w336 {
          tunnel: w335 -> [_ w367]
          tunnel: w334 -> [_ w366]
          tunnel: ["" w349] -> w333
          tunnel: w332 -> [_ w338]
          frame False {
          }
          frame True {
            w354 = "EnFlo_Tunnel:Chilled Water:Motor_Dem_Voltage"
            # "EnFlo_Tunnel:Chiller_Pump:Running"
            n137 = call "Read_value_of_earlier_Ch.vi"("Desired Ch to Read"="EnFlo_Tunnel:Chilled Water:Pressure_supply (Bar)", "Ch names"=w366, "Present scan array"=w367) -> ("Value"=w346:dbl, "Scan comment"=w353:string)  [unwired: 1 in]
            n138 = call "Read_value_of_earlier_Ch.vi"("Desired Ch to Read"="EnFlo_Tunnel:Chilled Water:Pressure_return (Bar)", "Ch names"=w366, "Present scan array"=w367) -> ("Value"=w362:dbl, "Scan comment"=w352:string)  [unwired: 1 in]
            n139 = call "Read_value_of_earlier_Ch.vi"("Desired Ch to Read"="EnFlo_Tunnel:Chilled Water:Desired_Delta_P", "Ch names"=w366, "Present scan array"=w367) -> ("Value"=w360:dbl, "Scan comment"=w351:string)  [unwired: 1 in]
            n140 = call "Read_value_of_earlier_Ch.vi"("Desired Ch to Read"=w354, "Ch names"=w366, "Present scan array"=w367) -> ("Value"=w343:dbl, "Scan comment"=w350:string)  [unwired: 1 in]
            n141 = Subtract(x=w346, y=w362) -> (x-y=w361:dbl)
            n142 = Subtract(x=w361, y=w360) -> (x-y=w355:dbl)
            n143 = Concatenate Strings(w353, w352, w351, w350) -> (w349:string)
            n144 = In Range and Coerce(upper limit=0.1 ("lower limit"), x=w355, lower limit=-0.1) -> (In Range?=w348:bool)  [unwired: 1 out]
            n145 = Less?(x=w346, y=3.85) -> (x < y?=w345:bool)
            n146 = Less?(x=w346, y=4.0) -> (x < y?=w356:bool)
            n147 = case shown="False" w338 {
              tunnel: w356 -> [_ w374]
              tunnel: w355 -> [_ w373]
              tunnel: w348 -> [_ w372]
              tunnel: w345 -> [_ w371]
              tunnel: w343 -> [_ w370]
              tunnel: [0.0 ("Value") w369] -> w340
              frame False {
              }
              frame True {
                n148 = case shown="True" w374 {
                  tunnel: w370 -> [w377 w380]
                  tunnel: w372 -> [_ w382]
                  tunnel: w373 -> [_ w381]
                  tunnel: [w375 w379] -> w369
                  tunnel: w371 -> [_ w378]
                  frame False {
                    n149 = Subtract(x=w377, y=0.2) -> (x-y=w375:dbl)
                  }
                  frame True {
                    n150 = case shown="False" w382 {
                      tunnel: w381 -> [w387 _]
                      tunnel: w380 -> [w386 w398]
                      tunnel: [w384 w398] -> w379
                      tunnel: w378 -> [w383 _]
                      frame False {
                        n151 = Greater Than 0?(x=w387) -> (x > 0?=w385:bool)
                        n152 = case shown="False" w385 {
                          tunnel: w386 -> [w389 w393]
                          tunnel: [w388 w392] -> w384
                          tunnel: w383 -> [_ w391]
                          frame True {
                            n153 = Subtract(x=w389, y=0.1) -> (x-y=w388:dbl)
                          }
                          frame False {
                            n154 = case shown="False" w391 {
                              tunnel: w393 -> [w394 w396]
                              tunnel: [w394 w395] -> w392
                              frame False {
                              }
                              frame True {
                                n155 = Add(x=w396, y=0.1) -> (x+y=w395:dbl)
                              }
                            }
                          }
                        }
                      }
                      frame True {
                      }
                    }
                  }
                }
              }
            }
            n156 = In Range and Coerce(upper limit=10.0, x=w340, lower limit=0.0) -> (coerced(x)=w339:dbl)  [unwired: 1 out]
            n157 = Equal?(x=w343, y=w339) -> (x = y?=w344:bool)
            n158 = case shown="False" w344 {
              tunnel: w354 -> [w400 _]
              tunnel: w339 -> [w399 _]
              frame False {
                n159 = Build Array(w400) -> (w401:string[])
                n160 = Build Array(w399) -> (w402:dbl[])
                n161 = call "ASYNC_Adam_server.vi"("Values"=w402, "Channel Names"=w401) -> ()  [unwired: 1 in, 3 out]
              }
              frame True {
              }
            }
          }
        }
      }
      frame #11 {
        n162 = while {
          tunnel: w405 -> [w421]
          tunnel: w404 -> [w420]
          shift-right: [w414] -> _
          shift-left: _ -> [w410]
          tunnel: [w406] -> w403
          stop <- FALSE continue-if-true
          w412 = 60.0 ("y")
          n163 = Decrement(x=w412) -> (x-1=w413:dbl)
          n164 = Select(t=w413, s=w410, f=w412) -> (s? t:f=w411:dbl)
          n165 = call "Read_value_of_earlier_Ch.vi"("Desired Ch to Read"="EnFlo_Tunnel:Chilled Water:Motor1 Temp", "Ch names"=w420, "Present scan array"=w421) -> ("Value"=w428:dbl, "Scan comment"=w408:string)  [unwired: 1 in]
          n166 = call "Read_value_of_earlier_Ch.vi"("Desired Ch to Read"="EnFlo_Tunnel:Chilled Water:Motor2 Temp", "Ch names"=w420, "Present scan array"=w421) -> ("Value"=w425:dbl, "Scan comment"=w407:string)  [unwired: 1 in]
          n167 = Greater?(x=w428, y=w411) -> (0:w422:bool)
          n168 = Greater?(x=w425, y=w411) -> (0:w423:bool)
          n169 = Or(x=w422, y=w423) -> (x .or. y?=w416:bool)
          n170 = call "Read_value_of_earlier_Ch.vi"("Desired Ch to Read"="EnFlo_Tunnel:Chiller_Pump:Enable", "Ch names"=w420, "Present scan array"=w421) -> ("Value"=w418:dbl, "Scan comment"=w409:string)  [unwired: 1 in]
          n171 = Greater?(x=w418, y=0.5) -> (0:w415:bool)
          n172 = And(x=w415, y=w416) -> (x .and. y?=w414:bool)
          n173 = Compound Arithmetic op=AND(w414, invert w410) -> (w427:bool)
          n174 = case shown="True" w427 {
            tunnel: w412 -> [_ w431]
            frame False {
            }
            frame True {
              n175 = Format Into String(format string="The Chilled Water Motor Temp is greater than %.0f deg C." ("Message"), w431) -> (resulting string=w430:string)  [unwired: 2 in, 1 out]
              n176 = call "Server_Emails.vi"("Client Name Contains"="EnFlo_Tunnel", "Message"=w430, "Subject"="Chilled Water Motor Temp") -> ()  [unwired: 2 in, 3 out]
            }
          }
          n177 = Concatenate Strings(w409, w408, w407) -> (w406:string)
        }
      }
      frame #12 {
        n178 = while {
          tunnel: w437 -> [w451]
          tunnel: w436 -> [w450]
          shift-right: [w439] -> _
          shift-left: _ -> [w445]
          shift-left: _ -> [w444]
          shift-left: _ -> [w443]
          tunnel: [w438] -> w435
          stop <- FALSE continue-if-true
          n179 = call "Read_value_of_earlier_Ch.vi"("Desired Ch to Read"="FFID:System:Enable", "Ch names"=w450, "Present scan array"=w451) -> ("Value"=w446:dbl, "Scan comment"=w438:string)  [unwired: 1 in]
          n180 = Greater?(x=w446, y=0.5) -> (0:w439:bool)
          n181 = Compound Arithmetic op=AND(w439, w445, invert w444, invert w443) -> (w441:bool)
          n182 = Compound Arithmetic op=AND(invert w439, invert w445, w444, w443) -> (w442:bool)
          n183 = Or(x=w441, y=w442) -> (x .or. y?=w440:bool)
          n184 = case shown="True" w440 {
            tunnel: w446 -> [_ w452]
            tunnel: w439 -> [_ _]
            frame False {
            }
            frame True {
              n185 = Build Array(w452) -> (w454:dbl[])
              n186 = call "ASYNC_Adam_server.vi"("Values"=w454, "Channel Names"=string[] ["GMU:Gas:Enable"]) -> ()  [unwired: 1 in, 3 out]
            }
          }
        }
      }
      frame #13 {
        n187 = Search 1D Array(1D array=w465, element="EnFlo_Tunnel:Motor:Enable" ("Desired Ch to Read")) -> (index of element=w462:i32)  [unwired: 1 out]
        n188 = Search 1D Array(1D array=w465, element="Status:of:EnFlo_Tunnel") -> (index of element=w470:i32)  [unwired: 1 out]
        n189 = Index Array(array=w463, index=w470) -> (element=w461:dbl)
        n190 = Index Array(array=w463, index=w462) -> (element=w460:dbl)
        n191 = To Long Integer(number=w461) -> (32bit integer=w456:i32)
        n192 = Greater?(x=w460, y=0.5) -> (0:w458:bool)
        n193 = case shown="0, Default" w456 {
          tunnel: [FALSE TRUE TRUE TRUE] -> w457
          frame 0, Default {
          }
          frame 1 {
          }
          frame 2 {
          }
          frame 3 {
          }
        }
        n194 = And(x=w457, y=w458) -> (x .and. y?=w455:bool)
        n195 = while {
          shift-right: [w482] -> _
          shift-left: _ -> [w483]
          tunnel: w455 -> [w482]
          tunnel: "EnFlo_Tunnel:Warning_Cone:Enable" -> [w484]
          tunnel: w467 -> [w479]
          tunnel: [w477] -> w466
          stop <- TRUE stop-if-true
          n196 = Not Equal?(x=w482, y=w483) -> (x != y?=w480:bool)
          n197 = Boolean To (0,1)(Boolean=w482) -> (0, 1=w476:i16)
          n198 = To Double Precision Float(number=w476) -> (double precision float=w475:dbl)
          n199 = Compound Arithmetic op=OR(w480, invert w479) -> (w478:bool)
          n200 = Build Array(w484) -> (w485:string[])
          n201 = Build Array(w475) -> (w486:dbl[])
          n202 = case shown="True" w478 {
            tunnel: w486 -> [_ w492]
            tunnel: w485 -> [_ w491]
            tunnel: ["" w488] -> w477
            frame False {
            }
            frame True {
              n203 = call "ASYNC_Adam_server.vi"("Values"=w492, "Channel Names"=w491) -> ("Scan Comments"=w489:string[])  [unwired: 1 in, 2 out]
              n204 = Index Array(array=w489, index=0) -> (element=w488:string)
            }
          }
        }
      }
      frame #14 {
        n205 = while {
          tunnel: w496 -> [w510]
          tunnel: w495 -> [w509]
          shift-right: [w497] -> _
          shift-left: _ -> [w504]
          shift-left: _ -> [w503]
          shift-left: _ -> [w502]
          tunnel: [w498] -> w494
          tunnel: [w497] -> w493
          stop <- FALSE continue-if-true
          n206 = call "Read_value_of_earlier_Ch.vi"("Desired Ch to Read"="EnFlo_Lab:Ventilation:Enable", "Ch names"=w509, "Present scan array"=w510) -> ("Value"=w505:dbl, "Scan comment"=w498:string)  [unwired: 1 in]
          n207 = Greater?(x=w505, y=0.5) -> (0:w497:bool)
          n208 = Compound Arithmetic op=AND(w497, w504, invert w503, invert w502) -> (w500:bool)
          n209 = Compound Arithmetic op=AND(invert w497, invert w504, w503, w502) -> (w501:bool)
          n210 = Or(x=w500, y=w501) -> (x .or. y?=w499:bool)
          n211 = case shown="True" w499 {
            tunnel: w505 -> [_ w511]
            frame False {
            }
            frame True {
              n212 = Build Array(1.0 ("element"), w511, w511) -> (w514:dbl[])
              n213 = call "ASYNC_Adam_server.vi"("Values"=w514, "Channel Names"=string[] ["EnFlo_Lab:Window:Enable", "EnFlo_Lab:Window:Open", "EnFlo_Lab:Window_Fans:Enable"]) -> ()  [unwired: 1 in, 3 out]
            }
          }
        }
      }
      frame #15 {
        n214 = while {
          shift-right: [w517] -> _
          shift-left: _ -> [w525]
          shift-left: _ -> [w524]
          shift-left: _ -> [w523]
          tunnel: w516 -> [w518]
          tunnel: w515 -> [w519]
          stop <- FALSE continue-if-true
          # "Opens the West window for ventilation if the EnFlo Tunnel is not measuring"
          n215 = Compound Arithmetic op=AND(w518, invert w519) -> (w517:bool)
          n216 = Compound Arithmetic op=AND(w517, w525, invert w524, invert w523) -> (w521:bool)
          n217 = Compound Arithmetic op=AND(invert w517, invert w525, w524, w523) -> (w522:bool)
          n218 = Or(x=w521, y=w522) -> (x .or. y?=w520:bool)
          n219 = case shown="True" w520 {
            tunnel: w517 -> [_ w527]
            frame False {
            }
            frame True {
              n220 = Select(t=1.0, s=w527, f=0.0) -> (s? t:f=w528:dbl)
              n221 = Build Array(w528, w528) -> (w532:dbl[])
              n222 = call "ASYNC_Adam_server.vi"("Values"=w532, "Channel Names"=string[] ["EnFlo_Lab:West Window:Open1", "EnFlo_Lab:West Window:Open2"]) -> ()  [unwired: 1 in, 3 out]
            }
          }
        }
      }
      frame #16 {
        n223 = while {
          tunnel: w537 -> [w549]
          tunnel: w536 -> [w548]
          shift-right: [w539] -> _
          shift-left: _ -> [w544]
          tunnel: [w543] -> w535
          tunnel: w534 -> [w541]
          tunnel: w533 -> [w538]
          stop <- FALSE continue-if-true
          w540 = "EnFlo_Tunnel:Motor:Enable" ("Desired Ch to Read")
          # "Re Zero EnFlo Tunnel static pressure when turning tunnel on"
          n224 = call "Read_value_of_earlier_Ch.vi"("Desired Ch to Read"=w540, "Ch names"=w548, "Present scan array"=w549) -> ("Value"=w545:dbl, "Scan comment"=w543:string)  [unwired: 1 in]
          n225 = Greater?(x=w545, y=0.5) -> (0:w539:bool)
          n226 = Compound Arithmetic op=AND(w539, invert w544, w538) -> (w542:bool)
          n227 = case shown="False" w542 {
            tunnel: w541 -> [_ w575]
            tunnel: w540 -> [_ w573]
            frame False {
            }
            frame True {
              w572 = "EnFlo_Tunnel:Pressure:Static"
              n228 = To Double Precision Float(number=w575) -> (double precision float=w558:dbl)
              n229 = Build Array(w572) -> (w571:string[])
              n230 = Build Array(w573, w572) -> (w576:string[])
              n231 = Subtract(x=w558, y=15.0) -> (x-y=w556:dbl)
              n232 = call "Get_Current_Scan_server.vi"("Desired Channels"=w571) -> ("Ch Description Array"=w570:T7[])  [unwired: 2 out]
              n233 = Subtract(x=w558, y=3600.0) -> (x-y=w574:dbl)
              n234 = call "Get_ADAM_averages_server.vi"("No of averages"=600, "End time"=w556, "Start time"=w574, "Clients time"=w558, "ADAM Ch Names"=w576) -> ("DBL values"=w560:dbl[][])  [unwired: 1 in, 4 out]
              n235 = Index Array(array=w570) -> (element=w568:T7)  [unwired: 1 in]
              n236 = Unbundle By Name(w568) -> ("A"=w569:dbl)
              n237 = Index Array(array=w560, index (col)=1 ("disabled index (col)")) -> (element=w555:dbl[])  [unwired: 1 in]
              n238 = Index Array(array=w560, index (col)=2 ("disabled index (col)")) -> (element=w554:dbl[])  [unwired: 1 in]
              n239 = Reverse 1D Array(array=w554) -> (reversed array=w550:dbl[])
              n240 = Reverse 1D Array(array=w555) -> (reversed array=w553:dbl[])
              n241 = for {
                tunnel: w553 -> [w578] mode=indexing
                tunnel: [w577] -> w552 mode=indexing
                tunnel: w550 -> [w577] mode=indexing
                stop <- w579 continue-if-true
                n242 = Less?(x=w578, y=0.01) -> (x < y?=w579:bool)
              }
              n243 = call "Mean_fr_NaN_data.vi"("Data"=w552) -> ("Mean value"=w551:dbl)  [unwired: 1 out]
              n244 = Subtract(x=w569, y=w551) -> (x-y=w567:dbl)
              n245 = Bundle By Name(cluster=w568, "A"=w567) -> (w566:T7)
              n246 = Build Array(w566) -> (w565:T7[])
              n247 = call "Update_Ch_Discription_server.vi"("Mode"=T3."Append to Global", "Channels to update In"=w565) -> ()  [unwired: 1 in, 1 out]
            }
          }
        }
      }
      frame #17 {
        # "Resetting A Tunnel speed to zero if the drive in turned off\nso that the belts do not slip when the tunnel is turned on again."
        n248 = while {
          tunnel: w584 -> [w597]
          tunnel: w583 -> [w596]
          shift-right: [w588] -> _
          shift-left: _ -> [w591]
          shift-left: _ -> [w590]
          shift-left: _ -> [w589]
          tunnel: w582 -> [w587]
          tunnel: [w585] -> w581
          stop <- FALSE continue-if-true
          n249 = call "Read_value_of_earlier_Ch.vi"("Desired Ch to Read"="A_Tunnel:Motor:Enable", "Ch names"=w596, "Present scan array"=w597) -> ("Value"=w592:dbl, "Scan comment"=w585:string)  [unwired: 1 in]
          n250 = Less?(x=w592, y=0.5) -> (x < y?=w588:bool)
          n251 = Compound Arithmetic op=AND(w588, w591, invert w590, invert w589, w587) -> (w586:bool)
          n252 = case shown="True" w586 {
            tunnel: w588 -> [_ _]
            frame False {
            }
            frame True {
              w600 = string[] ["A_Tunnel:Speed:Dem Velocity", "A_Tunnel:Speed:Dem Voltage"] ("Channel Names")
              n253 = Array Size(array=w600) -> (size(s)=w601:i32)
              n254 = Initialize Array(0.0 ("element"), w601) -> (w599:dbl[])
              n255 = call "ASYNC_Adam_server.vi"("Values"=w599, "Channel Names"=w600) -> ()  [unwired: 1 in, 3 out]
            }
          }
        }
      }
      frame #18 {
        # "Control Inlet fans"
        n256 = while {
          tunnel: w606 -> [w615]
          tunnel: w605 -> [w616]
          shift-right: [w607] -> w602
          shift-left: _ -> [w619]
          tunnel: w604 -> [w621]
          tunnel: [w612] -> w603
          stop <- FALSE continue-if-true
          n257 = call "Read_value_of_earlier_Ch.vi"("Desired Ch to Read"="EnFlo_Tunnel:Reference:Velocity", "Ch names"=w616, "Present scan array"=w615) -> ("Value"=w611:dbl, "Scan comment"=w613:string)  [unwired: 1 in]
          n258 = call "Read_value_of_earlier_Ch.vi"("Desired Ch to Read"="EnFlo_Tunnel:Motor:Enable", "Ch names"=w616, "Present scan array"=w615) -> ("Value"=w622:dbl, "Scan comment"=w614:string)  [unwired: 1 in]
          n259 = Greater?(x=w622, y=0.5) -> (0:w609:bool)
          n260 = Greater?(x=w611, y=0.15) -> (0:w608:bool)
          n261 = And(x=w608, y=w609) -> (x .and. y?=w607:bool)
          n262 = Not Equal?(x=w607, y=w619) -> (x != y?=w618:bool)
          n263 = Compound Arithmetic op=AND(w618, w621) -> (w620:bool)
          n264 = case shown="True" w620 {
            tunnel: w607 -> [_ w627]
            frame False {
            }
            frame True {
              n265 = case shown="True" w627 {
                tunnel: [string[] ["EnFlo_Tunnel:Inlet_Fans:Enable"] ("Channel Names") string[] ["EnFlo_Tunnel:Inlet_Fans:Enable", "Hydrosonic:Transducer:Setting"] ("Channel Names")] -> w629
                tunnel: [1.0 ("element") 0.0 ("element")] -> w626
                frame True {
                }
                frame False {
                }
              }
              n266 = Array Size(array=w629) -> (size(s)=w630:i32)
              n267 = Initialize Array(w626, w630) -> (w628:dbl[])
              n268 = call "ASYNC_Adam_server.vi"("Values"=w628, "Channel Names"=w629) -> ()  [unwired: 1 in, 3 out]
            }
          }
          n269 = Concatenate Strings(w613, w614) -> (w612:string)
        }
      }
      frame #19 {
        w646 = "EnFlo_Tunnel:Trav_Blockage_Fans:Demand_%"
        n270 = case shown="True" w641 {
          tunnel: w648 -> [_ w663]
          tunnel: w647 -> [_ w664]
          tunnel: w646 -> [_ w666]
          tunnel: [w653 w668] -> w642
          tunnel: ["" w659] -> w644
          tunnel: [w653 w655] -> w636
          frame False {
            w653 = 0.0 ("upper limit")
          }
          frame True {
            n271 = call "Read_value_of_earlier_Ch.vi"("Desired Ch to Read"="EnFlo_Tunnel:Trav_Blockage_Fans:Desired_Volts", "Ch names"=w664, "Present scan array"=w663) -> ("Value"=w658:dbl, "Scan comment"=w662:string)  [unwired: 1 in]
            n272 = call "Read_value_of_earlier_Ch.vi"("Desired Ch to Read"="EnFlo_Tunnel:Trav_Blockage_Fans:Meas_Volts", "Ch names"=w664, "Present scan array"=w663) -> ("Value"=w657:dbl, "Scan comment"=w661:string)  [unwired: 1 in]
            n273 = call "Read_value_of_earlier_Ch.vi"("Desired Ch to Read"=w666, "Ch names"=w664, "Present scan array"=w663) -> ("Value"=w655:dbl, "Scan comment"=w660:string)  [unwired: 1 in]
            n274 = Concatenate Strings(w662, w661, w660) -> (w659:string)
            n275 = call "Blockage_Fans_PID.vi"("Present Value"=w657, "Previous Control Sum"=w655, "Setpoint"=w658) -> ("Dem Output"=w656:dbl)
            n276 = In Range and Coerce(upper limit=100.0, x=w656, lower limit=0.0) -> (coerced(x)=w668:dbl)  [unwired: 1 out]
          }
        }
        n277 = Not Equal?(x=w642, y=w636) -> (x != y?=w638:bool)
        n278 = Compound Arithmetic op=OR(w638, invert w645) -> (w637:bool)
        n279 = Build Array(w646) -> (w639:string[])
        n280 = Build Array(w642) -> (w640:dbl[])
        n281 = case shown="True" w637 {
          tunnel: w640 -> [_ w652]
          tunnel: w639 -> [_ w651]
          tunnel: [string[] [] ("Scan Comments") w650] -> w643
          frame False {
          }
          frame True {
            n282 = call "ASYNC_Adam_server.vi"("Values"=w652, "Channel Names"=w651) -> ("Scan Comments"=w650:string[])  [unwired: 1 in, 2 out]
          }
        }
        n283 = Concatenate Strings(w644, w643) -> (w635:string)
      }
      frame #20 {
        # "Control Inlet fans"
        n284 = while {
          tunnel: w674 -> [w685]
          tunnel: w673 -> [w684]
          shift-right: [w675] -> _
          shift-left: _ -> [w676]
          tunnel: w672 -> [w679]
          tunnel: [w677] -> w671
          stop <- FALSE continue-if-true
          n285 = call "Read_value_of_earlier_Ch.vi"("Desired Ch to Read"="LDA:System:Enable", "Ch names"=w684, "Present scan array"=w685) -> ("Value"=w680:dbl, "Scan comment"=w677:string)  [unwired: 1 in]
          n286 = Greater?(x=w680, y=0.5) -> (0:w675:bool)
          n287 = Compound Arithmetic op=AND(w675, invert w676, w679) -> (w678:bool)
          n288 = case shown="True" w678 {
            tunnel: w675 -> [_ _]
            frame False {
            }
            frame True {
              w688 = string[] ["LDA1:Mains_Power:Enable"] ("Channel Names")
              n289 = Array Size(array=w688) -> (size(s)=w689:i32)
              n290 = Initialize Array(1.0 ("element"), w689) -> (w687:dbl[])
              n291 = call "ASYNC_Adam_server.vi"("Values"=w687, "Channel Names"=w688) -> ()  [unwired: 1 in, 3 out]
            }
          }
        }
      }
      frame #21 {
        n292 = And(x=w691, y=w692) -> (x .and. y?=w690:bool)
        n293 = case shown="False" w690 {
          tunnel: w695 -> [w700 _]
          tunnel: w694 -> [w699 _]
          tunnel: [w696 ""] -> w693
          frame False {
            n294 = for {
              tunnel: w700 -> [w710]
              tunnel: w699 -> [w709]
              tunnel: string[] ["EnFlo_Tunnel:Heater:Enable", "EnFlo_Tunnel:Chiller_Pump:Enable", "EnFlo_Tunnel:Tap_Water:Enable"] ("Ch Names") -> [w705] mode=indexing
              shift-right: [w703] -> w696
              shift-left: "" -> [w704]
              n295 = call "Read_value_of_earlier_Ch.vi"("Desired Ch to Read"=w705, "Ch names"=w709, "Present scan array"=w710) -> ("Value"=w707:dbl, "Scan comment"=w702:string)  [unwired: 1 in]
              n296 = Greater?(x=w707, y=0.5) -> (0:w706:bool)
              n297 = case shown="True" w706 {
                tunnel: w705 -> [_ w715]
                tunnel: ["" w712] -> w701
                frame False {
                }
                frame True {
                  n298 = Build Array(w715) -> (w718:string[])
                  n299 = Build Array(0.0) -> (w717:dbl[])
                  n300 = call "ASYNC_Adam_server.vi"("Values"=w717, "Channel Names"=w718) -> ("Scan Comments"=w713:string[])  [unwired: 1 in, 2 out]
                  n301 = Index Array(array=w713, index=0) -> (element=w712:string)
                }
              }
              n302 = Concatenate Strings(w704, w702, w701) -> (w703:string)
            }
          }
          frame True {
          }
        }
      }
      frame #22 {
        n303 = call "Read_value_of_earlier_Ch.vi"("Desired Ch to Read"="EnFlo_Tunnel:Reference:Velocity", "Ch names"=w725, "Present scan array"=w726) -> ("Value"=w728:dbl, "Scan comment"=w722:string)  [unwired: 1 in]
        n304 = Less?(x=w728, y=0.25) -> (x < y?=w727:bool)
        n305 = And(x=w720, y=w727) -> (x .and. y?=w724:bool)
        n306 = case shown="True" w724 {
          tunnel: ["" w733] -> w723
          frame False {
          }
          frame True {
            n307 = Build Array("EnFlo_Tunnel:Heater:Enable") -> (w738:string[])
            n308 = Build Array(0.0) -> (w737:dbl[])
            n309 = call "ASYNC_Adam_server.vi"("Values"=w737, "Channel Names"=w738) -> ("Scan Comments"=w734:string[])  [unwired: 1 in, 2 out]
            n310 = Index Array(array=w734, index=0) -> (element=w733:string)
          }
        }
        n311 = Concatenate Strings(w722, w723) -> (w721:string)
      }
      frame #23 {
        w740 = "EnFlo_Tunnel:Chiller_Pump_Floor:Dem_Power(%)" ("Ch Name")
        n312 = case shown="True" w741 {
          tunnel: w746 -> [_ w756]
          tunnel: w745 -> [_ w755]
          tunnel: [FALSE w753] -> w744
          tunnel: ["" w749] -> w742
          tunnel: w740 -> [_ w752]
          frame False {
          }
          frame True {
            n313 = call "Read_value_of_earlier_Ch.vi"("Desired Ch to Read"=w752, "Ch names"=w755, "Present scan array"=w756) -> ("Value"=w761:dbl, "Scan comment"=w751:string)  [unwired: 1 in]
            n314 = call "Read_value_of_earlier_Ch.vi"("Desired Ch to Read"="EnFlo_Tunnel:Floor_Cooling:Enable", "Ch names"=w755, "Present scan array"=w756) -> ("Value"=w758:dbl, "Scan comment"=w750:string)  [unwired: 1 in]
            n315 = Concatenate Strings(w751, w750) -> (w749:string)
            n316 = Greater?(x=w761, y=0.5) -> (0:w754:bool)
            n317 = Less?(x=w758, y=0.5) -> (x < y?=w757:bool)
            n318 = And(x=w754, y=w757) -> (x .and. y?=w753:bool)
          }
        }
        n319 = case shown="True" w744 {
          tunnel: ["" w765] -> w743
          tunnel: w740 -> [_ w764]
          frame False {
          }
          frame True {
            n320 = Build Array(0.0) -> (w769:dbl[])
            n321 = Build Array(w764) -> (w770:string[])
            n322 = call "ASYNC_Adam_server.vi"("Values"=w769, "Channel Names"=w770) -> ("Scan Comments"=w766:string[])  [unwired: 1 in, 2 out]
            n323 = Index Array(array=w766, index=0) -> (element=w765:string)
          }
        }
        n324 = Concatenate Strings(w742, w743) -> (w739:string)
      }
      frame #24 {
        n325 = call "Read_Earlier_Channels.vi"("Present scan array"=w777, "Ch names"=w778, "Desired Channels"=string[] ["Tank:Fill:Now", "Tank:Desired_Depth:mm", "Tank:Depth:mm", "Tank:Fill_Valve:Enable"]) -> ("Scan comments"=w785:string, "Index 0"=w791:dbl, "Index 1"=w788:dbl, "Index 2"=w787:dbl, "Index 3"=w789:dbl)  [unwired: 1 out]
        n326 = call "Read_value_of_earlier_Ch.vi"("Desired Ch to Read"="EnFlo Lab:Leak_Detector:Happy", "Ch names"=w778, "Present scan array"=w777) -> ("Value"=w775:dbl, "Scan comment"=w771:string)  [unwired: 1 in]
        n327 = Greater?(x=w791, y=0.5) -> (0:w774:bool)
        n328 = Greater?(x=w789, y=0.5) -> (0:w786:bool)
        n329 = Greater?(x=w775, y=0.5) -> (0:w772:bool)
        n330 = And(x=w772, y=w774) -> (x .and. y?=w773:bool)
        n331 = case shown="False" w773 {
          tunnel: w788 -> [_ w806]
          tunnel: w787 -> [_ w805]
          tunnel: w786 -> [w794 w801]
          tunnel: [w795 w803] -> w781
          tunnel: [w796 w802] -> w780
          frame False {
            n332 = case shown="True" w794 {
              tunnel: [dbl[] [] ("appended array") dbl[] [0.0] ("appended array")] -> w796
              tunnel: [string[] [] ("Desired Channels") string[] ["Tank:Fill_Valve:Enable"] ("Desired Channels")] -> w795
              frame False {
              }
              frame True {
                (unwired) "Tank:Fill_Valve:Enable"
              }
            }
          }
          frame True {
            n333 = Greater?(x=w806, y=w805) -> (0:w804:bool)
            n334 = case shown="True" w804 {
              tunnel: [string[] ["Tank:Fill:Now", "Tank:Fill_Valve:Enable"] ("Desired Channels") w811] -> w803
              tunnel: [dbl[] [0.0, 0.0] ("appended array") w810] -> w802
              tunnel: w801 -> [_ w809]
              frame False {
              }
              frame True {
                n335 = case shown="True" w809 {
                  tunnel: [string[] ["Tank:Fill_Valve:Enable"] ("Desired Channels") string[] [] ("Desired Channels")] -> w811
                  tunnel: [dbl[] [1.0] ("appended array") dbl[] [] ("appended array")] -> w810
                  frame False {
                    (unwired) "Tank:Fill_Valve:Enable"
                  }
                  frame True {
                  }
                }
              }
            }
          }
        }
        n336 = call "ASYNC_Adam_server.vi"("Values"=w780, "Channel Names"=w781) -> ("Scan Comments"=w782:string[])  [unwired: 1 in, 2 out]
        n337 = Concatenate Strings(w782) -> (w783:string)
        n338 = Concatenate Strings(w771, w783, w785) -> (w784:string)
      }
      frame #25 {
        n339 = call "Read_value_of_earlier_Ch.vi"("Desired Ch to Read"="EnFlo_Tunnel:Reference:Velocity", "Ch names"=w820, "Present scan array"=w821) -> ("Value"=w818:dbl, "Scan comment"=w816:string)  [unwired: 1 in]
        n340 = Greater?(x=w818, y=0.4) -> (0:w824:bool)
        n341 = Compound Arithmetic op=AND(w817, w824) -> (w822:bool)
      }
      frame #26 {
        w833 = "EnFlo_Tunnel:Heat_Ex_Div_Valve:Dem Pos"
        n342 = case shown="True" w834 {
          tunnel: w836 -> [_ w871]
          tunnel: w835 -> [_ w872]
          tunnel: w833 -> [_ w875]
          tunnel: [0.0 ("upper limit") w881] -> w825
          tunnel: ["" w866] -> w829
          frame False {
          }
          frame True {
            n343 = call "Read_value_of_earlier_Ch.vi"("Desired Ch to Read"="EnFlo_Tunnel:Exit Duct:Dem Temp", "Ch names"=w872, "Present scan array"=w871) -> ("Value"=w880:dbl, "Scan comment"=w870:string)  [unwired: 1 in]
            n344 = call "Read_value_of_earlier_Ch.vi"("Desired Ch to Read"="EnFlo_Tunnel:Exit Duct Top:Temp", "Ch names"=w872, "Present scan array"=w871) -> ("Value"=w876:dbl, "Scan comment"=w869:string)  [unwired: 1 in]
            n345 = call "Read_value_of_earlier_Ch.vi"("Desired Ch to Read"="EnFlo_Tunnel:Exit Duct:Temp", "Ch names"=w872, "Present scan array"=w871) -> ("Value"=w877:dbl, "Scan comment"=w868:string)  [unwired: 1 in]
            n346 = call "Read_value_of_earlier_Ch.vi"("Desired Ch to Read"=w875, "Ch names"=w872, "Present scan array"=w871) -> ("Value"=w878:dbl, "Scan comment"=w867:string)  [unwired: 1 in]
            n347 = Add(x=w876, y=w877) -> (x+y=w885:dbl)
            n348 = Divide(x=w885, y=2.0) -> (x/y=w887:dbl)
            n349 = Concatenate Strings(w870, w869, w868, w867) -> (w866:string)
            n350 = call "Back_End_Chiller_PID.vi"("Present Value"=w887, "Previous Control Sum"=w878, "Setpoint"=w880) -> ("Dem Output"=w884:dbl)
            n351 = In Range and Coerce(upper limit=100.0, x=w884, lower limit=0.0) -> (coerced(x)=w881:dbl)  [unwired: 1 out]
          }
        }
        n352 = case shown="False" w826 {
          tunnel: [w838 w849] -> w832
          tunnel: w825 -> [_ w849]
          tunnel: [w837 FALSE] -> w830
          frame False {
            # "Exercise valve once a week"
            n353 = Seconds To Date/Time() -> (date time rec=w839:T5)  [unwired: 2 out]
            n354 = Unbundle By Name(w839) -> ("day of week"=w844:i32, "hour"=w842:i32)
            n355 = Less?(x=w842, y=3) -> (x < y?=w847:bool)
            n356 = Equal?(x=7, y=w844) -> (x = y?=w846:bool)
            n357 = And(x=w846, y=w847) -> (x .and. y?=w837:bool)
            n358 = Select(t=100.0, s=w837, f=0.0) -> (s? t:f=w838:dbl)
          }
          frame True {
          }
        }
        n359 = while {
          shift-right: [w855] -> _
          shift-left: _ -> [w856]
          tunnel: w832 -> [w855]
          tunnel: w833 -> [w857]
          tunnel: w831 -> [w852]
          tunnel: [w850] -> w828
          stop <- TRUE stop-if-true
          n360 = Not Equal?(x=w855, y=w856) -> (x != y?=w853:bool)
          n361 = Compound Arithmetic op=OR(w853, invert w852) -> (w851:bool)
          n362 = Build Array(w857) -> (w858:string[])
          n363 = Build Array(w855) -> (w859:dbl[])
          n364 = case shown="True" w851 {
            tunnel: w859 -> [_ w863]
            tunnel: w858 -> [_ w862]
            tunnel: [string[] [] ("Scan Comments") w861] -> w850
            frame False {
            }
            frame True {
              n365 = call "ASYNC_Adam_server.vi"("Values"=w863, "Channel Names"=w862) -> ("Scan Comments"=w861:string[])  [unwired: 1 in, 2 out]
            }
          }
        }
        n366 = Concatenate Strings(w829, w828) -> (w827:string)
      }
      frame #27 {
        w891 = "EnFlo_Tunnel:Exit_Heaters:Dem_Power(%)"
        n367 = Equal To 0?(x=w902) -> (x = 0?=w900:bool)
        n368 = Greater?(x=w904, y=0.5) -> (0:w901:bool)
        n369 = And(x=w901, y=w900) -> (x .and. y?=w899:bool)
        n370 = case shown="True" w899 {
          tunnel: w890 -> [_ w920]
          tunnel: w889 -> [_ w919]
          tunnel: [0.0 w911] -> w898
          frame False {
          }
          frame True {
            n371 = call "Read_value_of_earlier_Ch.vi"("Desired Ch to Read"="EnFlo Lab:Heat:Extraction", "Ch names"=w919, "Present scan array"=w920) -> ("Value"=w917:dbl)  [unwired: 1 in, 1 out]
            n372 = Negate(x=w917) -> (-x=w916:dbl)
            n373 = In Range and Coerce(upper limit=12.0, x=w916, lower limit=0.0) -> (coerced(x)=w913:dbl)  [unwired: 1 out]
            n374 = Multiply(x=w913, y=8.33) -> (x*y=w911:dbl)
          }
        }
        n375 = call "Read_value_of_earlier_Ch.vi"("Desired Ch to Read"=w891, "Ch names"=w889, "Present scan array"=w890) -> ("Value"=w888:dbl)  [unwired: 1 in, 1 out]
        n376 = Not Equal?(x=w898, y=w888) -> (x != y?=w893:bool)
        n377 = Compound Arithmetic op=OR(w893, invert w897) -> (w892:bool)
        n378 = Build Array(w891) -> (w894:string[])
        n379 = Build Array(w898) -> (w895:dbl[])
        n380 = case shown="False" w892 {
          tunnel: w895 -> [_ w909]
          tunnel: w894 -> [_ w908]
          tunnel: ["" w906] -> w896
          frame False {
          }
          frame True {
            n381 = call "ASYNC_Adam_server.vi"("Values"=w909, "Channel Names"=w908) -> ("Scan Comments"=w907:string[])  [unwired: 1 in, 2 out]
            n382 = Index Array(array=w907) -> (element=w906:string)  [unwired: 1 in]
          }
        }
      }
      frame #28 {
        # "Only starts to run the back end Chiller boost Pump when the EnFlo_Tunnel:Heat_Ex_Div_Valve:Dem Pos\nis more than 75%"
        n383 = Greater?(x=w921, y=75.0) -> (0:w924:bool)
        n384 = Greater?(x=w931, y=0.5) -> (0:w925:bool)
        n385 = And(x=w925, y=w924) -> (x .and. y?=w923:bool)
        n386 = case shown="True" w923 {
          tunnel: [0.0 w948] -> w929
          tunnel: w921 -> [_ w954]
          frame False {
          }
          frame True {
            n387 = Subtract(x=w954, y=50.0) -> (x-y=w952:dbl)
            n388 = Quotient & Remainder(x=w952, y=10.0) -> (floor(x/y)=w950:dbl)  [unwired: 1 out]
            n389 = Multiply(x=w950, y=20.0) -> (x*y=w948:dbl)
          }
        }
        n390 = while {
          shift-right: [w937] -> _
          shift-left: _ -> [w938]
          tunnel: w929 -> [w937]
          tunnel: "EnFlo_Tunnel:Chiller_Pump_Exchanger:Dem_Power(%)" -> [w939]
          tunnel: w927 -> [w934]
          tunnel: [w932] -> w922
          stop <- TRUE stop-if-true
          n391 = Not Equal?(x=w937, y=w938) -> (x != y?=w935:bool)
          n392 = Compound Arithmetic op=OR(w935, invert w934) -> (w933:bool)
          n393 = Build Array(w939) -> (w940:string[])
          n394 = Build Array(w937) -> (w941:dbl[])
          n395 = case shown="False" w933 {
            tunnel: w941 -> [_ w946]
            tunnel: w940 -> [_ w945]
            tunnel: ["" w943] -> w932
            frame False {
            }
            frame True {
              n396 = call "ASYNC_Adam_server.vi"("Values"=w946, "Channel Names"=w945) -> ("Scan Comments"=w944:string[])  [unwired: 1 in, 2 out]
              n397 = Index Array(array=w944) -> (element=w943:string)  [unwired: 1 in]
            }
          }
        }
      }
      frame #29 {
        n398 = while {
          shift-right: [w962] -> _
          shift-left: _ -> [w963]
          tunnel: w957 -> [w962]
          tunnel: [w959] -> w956
          tunnel: w955 -> [w958]
          stop <- TRUE stop-if-true
          n399 = Compound Arithmetic op=AND(w958, invert w963, w962) -> (w960:bool)
          n400 = case shown="True" w960 {
            tunnel: ["" w966] -> w959
            frame False {
            }
            frame True {
              n401 = Build Array("EnFlo Lab:Heat:Extraction") -> (w971:string[])
              n402 = Build Array(0.0) -> (w970:dbl[])
              n403 = call "ASYNC_Adam_server.vi"("Values"=w970, "Channel Names"=w971) -> ("Scan Comments"=w967:string[])  [unwired: 1 in, 2 out]
              n404 = Index Array(array=w967, index=0) -> (element=w966:string)
            }
          }
        }
      }
      frame #30 {
        # "To automatically control the request for the University Stall chiller to run."
        n405 = while {
          tunnel: w976 -> [w990]
          tunnel: w975 -> [w991]
          shift-right: [w983] -> _
          shift-left: _ -> [w1000]
          shift-left: _ -> [w999]
          shift-left: _ -> [w998]
          tunnel: [w989] -> w974
          tunnel: [w988] -> w973
          stop <- FALSE continue-if-true
          n406 = Build Array("Aero_Tunnel:Cooling_Pump:Enable" ("Desired Ch to Read"), "EnFlo_Tunnel:Chiller_Pump:Enable" ("Desired Ch to Read"), "EnFlo_Tunnel:Chilled Water:Motor_Dem_Voltage" ("Desired Ch to Read")) -> (w992:string[])
          n407 = call "Read_Earlier_Channels.vi"("Present scan array"=w990, "Ch names"=w991, "Desired Channels"=w992) -> ("Scan comments"=w988:string, "Index 0"=w986:dbl, "Index 1"=w982:dbl, "Index 2"=w981:dbl)  [unwired: 2 out]
          n408 = Greater?(x=w986, y=0.5) -> (0:w977:bool)
          n409 = Greater?(x=w981, y=0.1) -> (0:w979:bool)
          n410 = Greater?(x=w982, y=0.5) -> (0:w980:bool)
          n411 = And(x=w980, y=w979) -> (x .and. y?=w978:bool)
          n412 = Or(x=w977, y=w978) -> (x .or. y?=w983:bool)
          n413 = Compound Arithmetic op=AND(w983, w1000, invert w999, invert w998) -> (w996:bool)
          n414 = Compound Arithmetic op=AND(invert w983, invert w1000, w999, w998) -> (w997:bool)
          n415 = Or(x=w996, y=w997) -> (x .or. y?=w995:bool)
          n416 = case shown="True" w995 {
            tunnel: w983 -> [_ w1009]
            tunnel: [string[] [] ("Scan Comments") w1004] -> w989
            frame False {
            }
            frame True {
              n417 = case shown="True" w1009 {
                tunnel: [string[] ["University:Chilled Water:Requested"] ("Channel Names") string[] ["University:Chilled Water:Requested"] ("Channel Names")] -> w1008
                tunnel: [1.0 ("y") 0.0 ("y")] -> w1005
                frame True {
                }
                frame False {
                }
              }
              n418 = Array Size(array=w1008) -> (size(s)=w1006:i32)
              n419 = Initialize Array(w1005, w1006) -> (w1007:dbl[])
              n420 = call "ASYNC_Adam_server.vi"("Values"=w1007, "Channel Names"=w1008) -> ("Scan Comments"=w1004:string[])  [unwired: 1 in, 2 out]
            }
          }
        }
        n421 = Concatenate Strings(w974, w973) -> (w972:string)
      }
      frame #31 {
        # "Exercise the floor cooling valve once a week"
        n422 = while {
          shift-right: [w1018] -> _
          shift-left: _ -> [w1023]
          tunnel: w1016 -> [w1018]
          tunnel: w1015 -> [w1020]
          tunnel: [w1017] -> w1014
          stop <- TRUE stop-if-true
          n423 = Not Equal?(x=w1018, y=w1023) -> (x != y?=w1021:bool)
          n424 = Compound Arithmetic op=AND(w1021, w1020) -> (w1019:bool)
          n425 = case shown="True" w1019 {
            tunnel: w1018 -> [_ w1030]
            tunnel: ["" w1025] -> w1017
            frame False {
            }
            frame True {
              n426 = Select(t=1.0, s=w1030, f=0.0) -> (s? t:f=w1031:dbl)
              n427 = Build Array(w1031) -> (w1034:dbl[])
              n428 = Build Array("EnFlo_Tunnel:Floor_Cooling:Enable") -> (w1033:string[])
              n429 = call "ASYNC_Adam_server.vi"("Values"=w1034, "Channel Names"=w1033) -> ("Scan Comments"=w1026:string[])  [unwired: 1 in, 2 out]
              n430 = Index Array(array=w1026, index=0) -> (element=w1025:string)
            }
          }
        }
      }
      frame #32 {
        n431 = Build Array("GMU:CO2_Low:Siren") -> (w1039:string[])
        n432 = Quotient & Remainder(x=w1052, y=15) -> (x-y*floor(x/y)=w1050:i32)  [unwired: 1 out]
        n433 = call "Get_Current_Scan_server.vi"("Desired Channels"=w1039) -> ("Ch Description Array"=w1056:T7[], "Numerical Values"=w1046:dbl[])  [unwired: 1 out]
        n434 = Equal To 0?(x=w1050) -> (x = 0?=w1049:bool)
        n435 = Select(t=1.0, s=w1049, f=0.0) -> (s? t:f=w1048:dbl)
        n436 = Index Array(array=w1056, index=0) -> (element=w1055:T7)
        n437 = Index Array(array=w1046, index=0) -> (element=w1035:dbl)
        n438 = Unbundle By Name(w1055) -> ("A"=w1054:dbl)
        n439 = Greater?(x=w1035, y=0.5) -> (0:w1042:bool)
        n440 = Greater?(x=w1054, y=0.5) -> (0:w1043:bool)
        n441 = Not Equal?(x=w1048, y=w1035) -> (x != y?=w1037:bool)
        n442 = Or(x=w1043, y=w1042) -> (x .or. y?=w1041:bool)
        n443 = Build Array(w1048) -> (w1038:dbl[])
        n444 = Compound Arithmetic op=AND(w1037, w1041) -> (w1036:bool)
        n445 = case shown="True" w1036 {
          tunnel: w1038 -> [_ w1065]
          tunnel: w1039 -> [_ w1064]
          tunnel: ["" w1061] -> w1040
          frame False {
          }
          frame True {
            n446 = call "ASYNC_Adam_server.vi"("Values"=w1065, "Channel Names"=w1064) -> ("Scan Comments"=w1062:string[])  [unwired: 1 in, 2 out]
            n447 = Index Array(array=w1062, index=0) -> (element=w1061:string)
          }
        }
      }
      frame #33 {
        n448 = Concatenate Strings(w1066, w1067, w1068, w1069, w1070, w1072, w1071, w1073, w1074, w1075, w1076, w1077, w1083, w1084, w1085, w1086, w1087, w1088, w1089, w1096, w1095, w1094, w1093, w1092, w1091, w1090, w1081, w1080, w1079, w1078) -> (→"Scan comment":string)
      }
    }
  }
